vi "Dashboard Main.vi"() -> ()   [LabVIEW 2017]
uses:
  <vilib>/Utility/miscctls.llb/LVRowAndColumnTypeDef.ctl
  <vilib>/event_ctls.llb/eventvkey.ctl
  <vilib>/Rock Robotics/Network Tables/NT Read Boolean.vi
  <vilib>/Rock Robotics/Network Tables/NT Write Boolean.vi
  <vilib>/Rock Robotics/WPI/Dashboard/WPI_DashboardLogging Global.vi
panel:
  out "Camera Image":T1(plugin-control)
  out "Camera Info":cluster{"Mbps LED":bool, "Mbps":dbl, "fps":dbl} {"fps" format="%#.1g"; "Mbps" format="%#.1g"}
  in  "Camera Name":string(combo)="No Camera Selection"
  in  "Camera Settings":T2={"Frame Rate"=30, "Compression"=30, "Size"=1, "DB Camera Config"=FALSE} {"Frame Rate" scale=1.0..30.0; "Compression" scale=100.0..-1.0; "Size" items=["640x480", "320x240", "160x120"]}
  out "Camera Image Right":T1(plugin-control)
  out "NT Connection":bool
  in  "Camera Settings Right":T2={"Frame Rate"=30, "Compression"=30, "Size"=1, "DB Camera Config"=FALSE} {"Frame Rate" scale=1.0..30.0; "Compression" scale=100.0..-1.0; "Size" items=["640x480", "320x240", "160x120"]}
  in  "Camera Name Right":string(combo)="No Camera Selection"
  in  "TCP":refnum<k5>
  in  "Rec Mode":enum32{"Stop", "Record", "Playback"}(radio)
  out "Robot IP":string
  out "Image Message":string="Timeout in Camera Communications"
  in  "Dashboard Tab":T3(tab)
  out "RPED":enum32{"Read", "Write"}(tab)=enum."Write"
  out "Current Left Backward Power":dbl
  out "Current Right Backward Power":dbl
  out "Current Left Forward Power":dbl
  out "Current Right Forward Power":dbl
  in  "Right Backward Power":dbl
  in  "Left Backward Power":dbl
  in  "Right Forward Power":dbl
  in  "Left Forward Power":dbl
  out "Lift":enum32{"Read", "Write"}(tab)=enum."Write"
  out "Current Exchange Encoder Position":dbl
  out "Current Climb Power":dbl
  out "Current Manual Up Power":dbl
  out "Current Manual Down Power":dbl
  out "Current Scale High Encoder Position":dbl
  out "Current Scale Mid Encoder Position":dbl
  out "Current Scale Low Encoder Position":dbl
  out "Current Switch Encoder Position":dbl
  out "Current Stow Encoder Position":dbl
  out "Current Climb Encoder Position":dbl
  out "Current Load Encoder Position":dbl
  out "Current Portal Encoder Position":dbl
  in  "Portal Encoder Position":dbl
  in  "Exchange Encoder Position":dbl
  in  "Climb Power":dbl
  in  "Manual Up Power":dbl
  in  "Manual Down Power":dbl
  in  "Scale High Encoder Position":dbl
  in  "Scale Low Encoder Position":dbl
  in  "Scale Mid Encoder Position":dbl
  in  "Climb Encoder Position":dbl
  in  "Switch Encoder Position":dbl
  in  "Stow Encoder Position":dbl
  in  "Load Encoder Position":dbl
  out "Intake Rotation":enum32{"Read", "Write"}(tab)=enum."Write"
  out "Current Intake Rot Portal Encoder Position":dbl
  out "Current Intake Rot Exchange Encoder Position":dbl
  out "Current Intake Rot Climb Encoder Position":dbl
  out "Current Intake Rot Switch Encoder Position":dbl
  out "Current Intake Rot Stow Encoder Position":dbl
  out "Current Intake Rot Scale High Encoder Position":dbl
  out "Current Intake Rot Load Encoder Position":dbl
  out "Current Intake Rot Manual Down Power":dbl
  out "Current Intake Rot Manual Up Power":dbl
  out "Current Intake Rot Scale Mid Encoder Position":dbl
  out "Current Intake Rot Scale Low Encoder Position":dbl
  in  "Intake Rot Portal Encoder Position":dbl
  in  "Intake Rot Exchange Encoder Position":dbl
  in  "Intake Rot Climb Encoder Positon":dbl
  in  "Intake Rot Switch Encoder Position":dbl
  in  "Intake Rot Stow Encoder Position":dbl
  in  "Intake Rot Scale High Encoder Position":dbl
  in  "Intake Rot Load Encoder Position":dbl
  in  "Intake Rot Manual Up Power":dbl
  in  "Intake Rot Manual Down Power":dbl
  in  "Intake Rot Scale Mid Encoder Position":dbl
  in  "Intake Rot Scale Low Encoder Position":dbl
  out "Drive":enum32{"Read", "Write"}(tab)=enum."Write"
  out "Current Right Low Gear P":dbl
  out "Current Right Low Gear I":dbl
  out "Current Right Low Gear D":dbl
  out "Current Right Low Gear F":dbl
  out "Current Right High Gear I":dbl
  out "Current Right High Gear P":dbl
  out "Current Right High Gear D":dbl
  out "Current Right High Gear F":dbl
  out "Current Left Low Gear P":dbl
  out "Current Left Low Gear I":dbl
  out "Current Left Low Gear D":dbl
  out "Current Left Low Gear F":dbl
  out "Current Left High Gear I":dbl
  out "Current Left High Gear P":dbl
  out "Current Left High Gear D":dbl
  out "Current Left High Gear F":dbl
  in  "Right High Gear F":dbl
  in  "Right High Gear D":dbl
  in  "Right High Gear I":dbl
  in  "Right High Gear P":dbl
  in  "Right  Low Gear F":dbl
  in  "Right Low Gear D":dbl
  in  "Right Low Gear I":dbl
  in  "Right Low Gear P":dbl
  in  "Left High Gear F":dbl
  in  "Left High Gear D":dbl
  in  "Left High Gear I":dbl
  in  "Left High Gear P":dbl
  in  "Left Low Gear F":dbl
  in  "Left Low Gear D":dbl
  in  "Left Low Gear I":dbl
  in  "Left Low Gear P":dbl
  out "Left Wheel":dbl
  out "Right Wheel":dbl
  out "Lift Upper Switch":bool
  out "Arm Lower Switch":bool
  out "IMU":dbl(knob) scale=-360.0..360.0
  out "Last Auto Play Run":string
  out "Brake":bool
  out "Arm":bool
  out "Has Cube":bool
  out "Lift Position":dbl(slide) scale=0.0..7.0
  out "Arm Encoder Position":dbl
  out "Arm Stowed":bool
  out "Lift Stowed":bool
  out "Mode":T4(ring)=enum."Auto Disabled"
  out "Match Time":string="0:00"
  out "High Gear":bool
  out "Lift Encoder Position":dbl
  in  "Override":enum16{"Default", "LL", "LR", "RL", "RR"}(ring)
  in  "RL":T5(ring)
  in  "RR":T6(ring)
  in  "LR":T5(ring)
  in  "LL":T7(ring)
  in  "Position":enum16{"1", "2", "3"}(ring)
  out "Auto":enum32{"Read", "Write"}(tab)
  out "Current Cube PID Acceptable Error":dbl
  out "Current Turning Acceptable Error":dbl
  out "Current Turning Acceptable Tolerance":dbl
  out "Current Number of Loops to be in Tolerance":dbl
  out "Current Number of Loops to be in Acceptable Error":dbl
  out "Current Kp Lower":dbl
  out "Current Kd Lower":dbl
  out "Current Ki Lower":dbl
  out "Current Cube P":dbl
  out "Current Cube D":dbl
  out "Current Cube I":dbl
  out "Current Turn Distance I":dbl
  out "Current Turn Distance P":dbl
  out "Current Kp Upper":dbl
  out "Current Turn Distance D":dbl
  out "Current Kd Upper":dbl
  out "Current Ki Upper":dbl
  in  "Cube PID Acceptable Error":dbl
  in  "Turning Acceptable Error":dbl
  in  "Turning Acceptable Tolerance":dbl
  in  "Number of Loops to be in Acceptable Error":dbl
  in  "Number of Loops to be in Tolerance":dbl
  in  "Kp Lower":dbl
  in  "Ki Lower":dbl
  in  "Kd Lower":dbl
  in  "Turn Distance P":dbl
  in  "Turn Distance I":dbl
  in  "Turn Distance D":dbl
  in  "Kp Upper":dbl
  in  "Ki Upper":dbl
  in  "Kd Upper":dbl
  in  "Cube I":dbl
  in  "Cube D":dbl
  in  "Cube P":dbl
  in  "DB/String 9":string
  in  "DB/String 8":string
  in  "DB/String 7":string
  in  "DB/String 6":string
  in  "DB/String 5":string
  in  "DB/String 4":string
  in  "DB/String 3":string
  in  "DB/String 2":string
  in  "DB/String 1":string
  in  "DB/String 0":string
  in  "DB/Slider 0":dbl(slide) scale=0.0..5.0
  in  "DB/Slider 1":dbl(slide) scale=0.0..5.0
  in  "DB/Slider 2":dbl(slide) scale=0.0..5.0
  in  "DB/Slider 3":dbl(slide) scale=0.0..5.0
  out "DB/LED 3":bool
  out "DB/LED 2":bool
  out "DB/LED 1":bool
  out "DB/LED 0":bool
  in  "DB/Button 3":bool
  in  "DB/Button 2":bool
  in  "DB/Button 1":bool
  in  "DB/Button 0":bool caption="New Name"
  in  "Test Slider":dbl(slide) scale=0.0..100.0 scale format="%#_3g"
  in  "On/Off":bool caption="Solenoid"
  in  "Test Name":u16(ring) items=["Select the test to run..."]
  in  "Test Tree":string(tree)
  in  "Motor":cluster{"Value":dbl, "Enable":bool} {"Value" scale=-1.0..1.0 scale format="%#_3g"}
  out "Progress":T8 {"Test Progress" scale=0.0..100.0}
  in  "Rev/Fwd":cluster{"Forward":bool, "Reverse":bool}
  in  "Test Ring":u16(ring) items=["Monochrome", "Color"]
  out "Cmd Status":string
  in  "Execute Command":bool
  in  "Command Params":string[][](table)
  in  "Command Selection":i32(listbox)
  in  "CheckList":i32(listbox)
  out "Tree":string(tree)
  out "Background":bool
  # "HW"
  # "HW"
  # "Pnuematics"
  # "Turning"
  # "Cube"
  # "Turning"
  # "Cube"
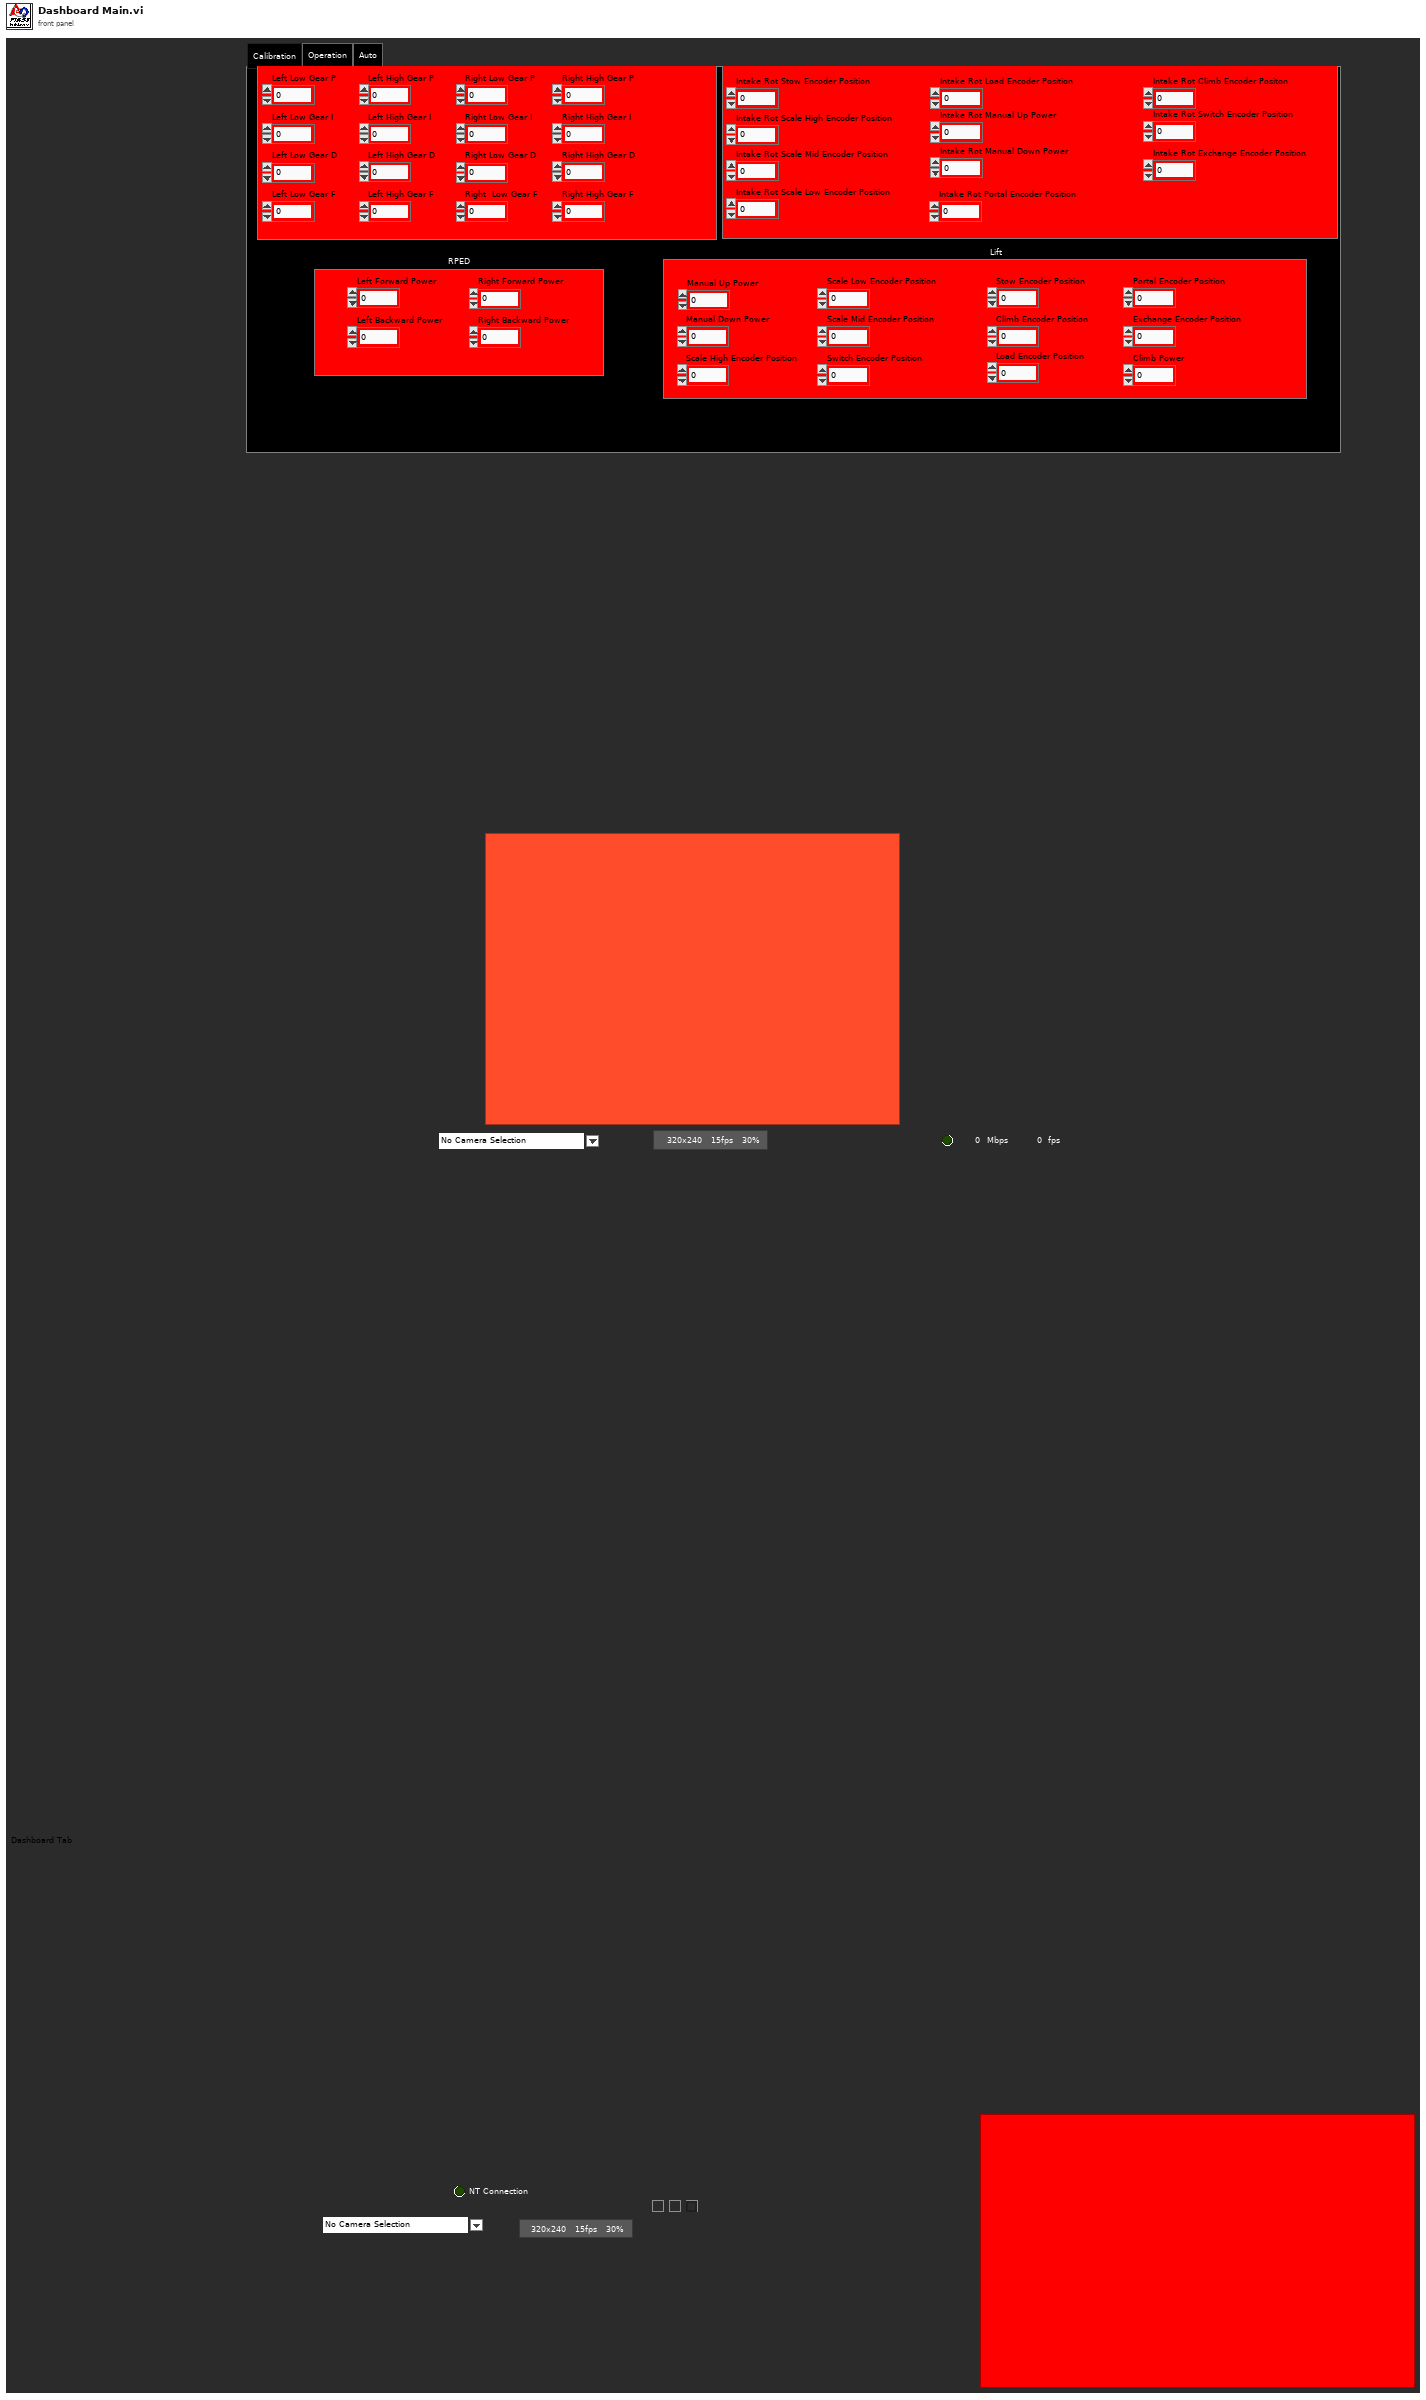
[diagram p1: front panel]
types:
  T1 = typedef "IMAQ Image.ctl" = refnum<image>
  T2 = cluster{"Frame Rate":i32, "Compression":i32, "Size":u16, "DB Camera Config":bool}
  T3 = enum32{"Calibration", "Operation", "Auto", "Basic", "Custom", "Test", "Commands", "Checklist", "Variables"}
  T4 = enum8{"Tele-Op Disabled", "Tele-Op Enabled", "Auto Disabled", "Auto Enabled", "Test Disabled", "Test Enabled", "Disconnected", "No Code", "E-Stop"}
  T5 = enum16{"No_Op", "Auto_Run_Backwards", "Auto_Run_Forwards", "Switch", "Switch_2", "Scale", "Adapt_Scale", "Scale_2", "Switch_Scale", "Scale_Drop_Cube"}
  T6 = enum16{"No_Op", "Auto_Run_Forwards", "Auto_Run_Backwards", "Switch", "Switch_2", "Scale", "Adapt_Scale", "Switch_Scale", "Scale_Switch", "Scale_2", "Drop_Pickup"}
  T7 = enum16{"No_Op", "Auto_Run_Backwards", "Auto_Run_Forwards", "Switch", "Switch_2", "Scale", "Adapt_Scale", "Switch_Scale", "Scale_Switch", "Scale_2", "Drop_Pickup"}
  T8 = cluster{"Test Progress":u8, "Test Progress Text":string}
  T9 = cluster{"Save Path":path, "Interval (s)":dbl, "Keep":i32}
  T10 = enum32{"Drive", "Camera", "Basic", "Custom", "Test", "Commands", "Checklist", "Variables"}
  T11 = typedef "Image Type" = u32
  T12 = cluster{"IDs":cluster{"RPC field ID":u16, "Unique ID":u16}, "String":string}
  T13 = cluster{"Error Strings":string, "Disable Counts":cluster{u16, u16}, "Rail Faults":cluster{u16, u16, u16}, "Robot IP":string, "DB Mode":u8, "Event Info":cluster{"Name":string, "Type":u8, "Number":u16, "Replay":u8}}
  T14 = cluster{"Storage":cluster{"Disk Free":u64, "RAM Block":u32, "RAM free":u32}, "CPU Utilization":cluster{"CPU % ISR":sgl, "CPU % Time Crit":sgl, "CPU % Timed Str":sgl, "CPU % High":sgl, "CPU % Above":sgl, "CPU % Normal":sgl, "CPU % Low":sgl}, "CAN":cluster{"% Bus Utilization":sgl, "Bus Off Cnt":u32, "TX_FIFO Full Cnt":u32, "Receive Error Cnt":u8, "Transmit Error Cnt":u8}, "HID":cluster{"HID Outputs":u32, "Rumble Low":u16, "Rumble High":u16}[]}
  T15 = cluster{"Status bits":cluster{"Test Mode":bool, "Autonomous":bool, "Enabled":bool, "Code Start":bool, "Brownout":bool, "Reserved 2":bool, "Reserved 3":bool, "E-Stop":bool}, "Code Trace":cluster{"Disabled":bool, "TeleOp":bool, "Auto":bool, "Test":bool}, "Controller Type":enum16{"unknown", "cRIO", "roboRio"}, "Code?":enum16{"unknown", "noCode", "code"}, "Battery V":dbl}
  T16 = cluster{"Control Bits":cluster{"TestMode":bool, "Autonomous":bool, "Enabled":bool, "FMS Present":bool, bool, bool, bool, "E-Stop":bool}, "Team Station ":u8, "Countdown":sgl, "Joystick Values":cluster{"Axes":dbl[], "Buttons":bool[], "POVs":i16[]}[]}
  T17 = cluster{"Camera Image":refnum<vi>, "Dashboard Tab":refnum<vi>, "Background":refnum<vi>, "Rec Mode":refnum<vi>, "Test Slider":refnum<vi>, "On/Off ":refnum<vi>, "Test Ring":refnum<vi>, "Rev/Fwd":refnum<vi>, "Test Name":refnum<vi>, "Motor":refnum<vi>, "Progress":refnum<vi>, "CheckList":refnum<vi>, "Tree":refnum<vi>, "Test Tree":refnum<vi>, "Command Params":refnum<vi>, "Command Selection":refnum<vi>, "Execute Command":refnum<vi>, "Cmd Status":refnum<vi>, "Camera Settings":refnum<vi>, "Camera Name":refnum<vi>, "Camera Info":refnum<vi>, "Camera Settings Right":refnum<vi>, "Camera Name Right":refnum<vi>, "Camera Image Right":refnum<vi>}
  T18 = cluster{"Camera Name Right":string, string, "Saved DB Images Info":cluster{"Save Path":path, "Interval (s)":dbl, "Keep":i32}}
  T19 = cluster{"Camera Name":string, string, "Saved DB Images Info":cluster{"Save Path":path, "Interval (s)":dbl, "Keep":i32}}
  T20 = cluster{"Operation":enum16{"Update", "Clear"}, "Color Box":u32}[]
  T21 = typedef "eventvkey.ctl" = enum16{"ASCII", "Enter", "Return", "Shift", "Ctrl", "Alt", "Cmd", "Opt", "Caps", "NumLock", "Clear", "Break", "Up", "Down", "Left", "Right", "Insert", "Delete", "Home", "End", "PageUp", "PageDown", "Escape", "Help", "Pause", "ScrollLock", "F1", "F2", "F3", "F4", "F5", "F6", "F7", "F8", "F9", "F10", "F11", "F12", "F13", "F14", "F15", "F16", "F17", "F18", "F19", "F20", "F21", "F22", "F23", "F24", "Play", "VolumeUp", "VolumeDown", "Mute", "Two Byte Char"}
  T22 = cluster{"Image Size":bool, "Image Type":bool, "Pixel Value":bool, "ROI Information":bool, "Zoom Factor":bool}
  T23 = cluster{"Operation":enum16{"Update", "Clear"}, "Color Box":u32}
  T24 = typedef "LVRowAndColumnTypeDef.ctl" = cluster{"Row":i32, "Column":i32}
  T25 = cluster{"Shift":bool, "Ctrl":bool, "Alt":bool, "Cmd":bool, "Opt":bool}
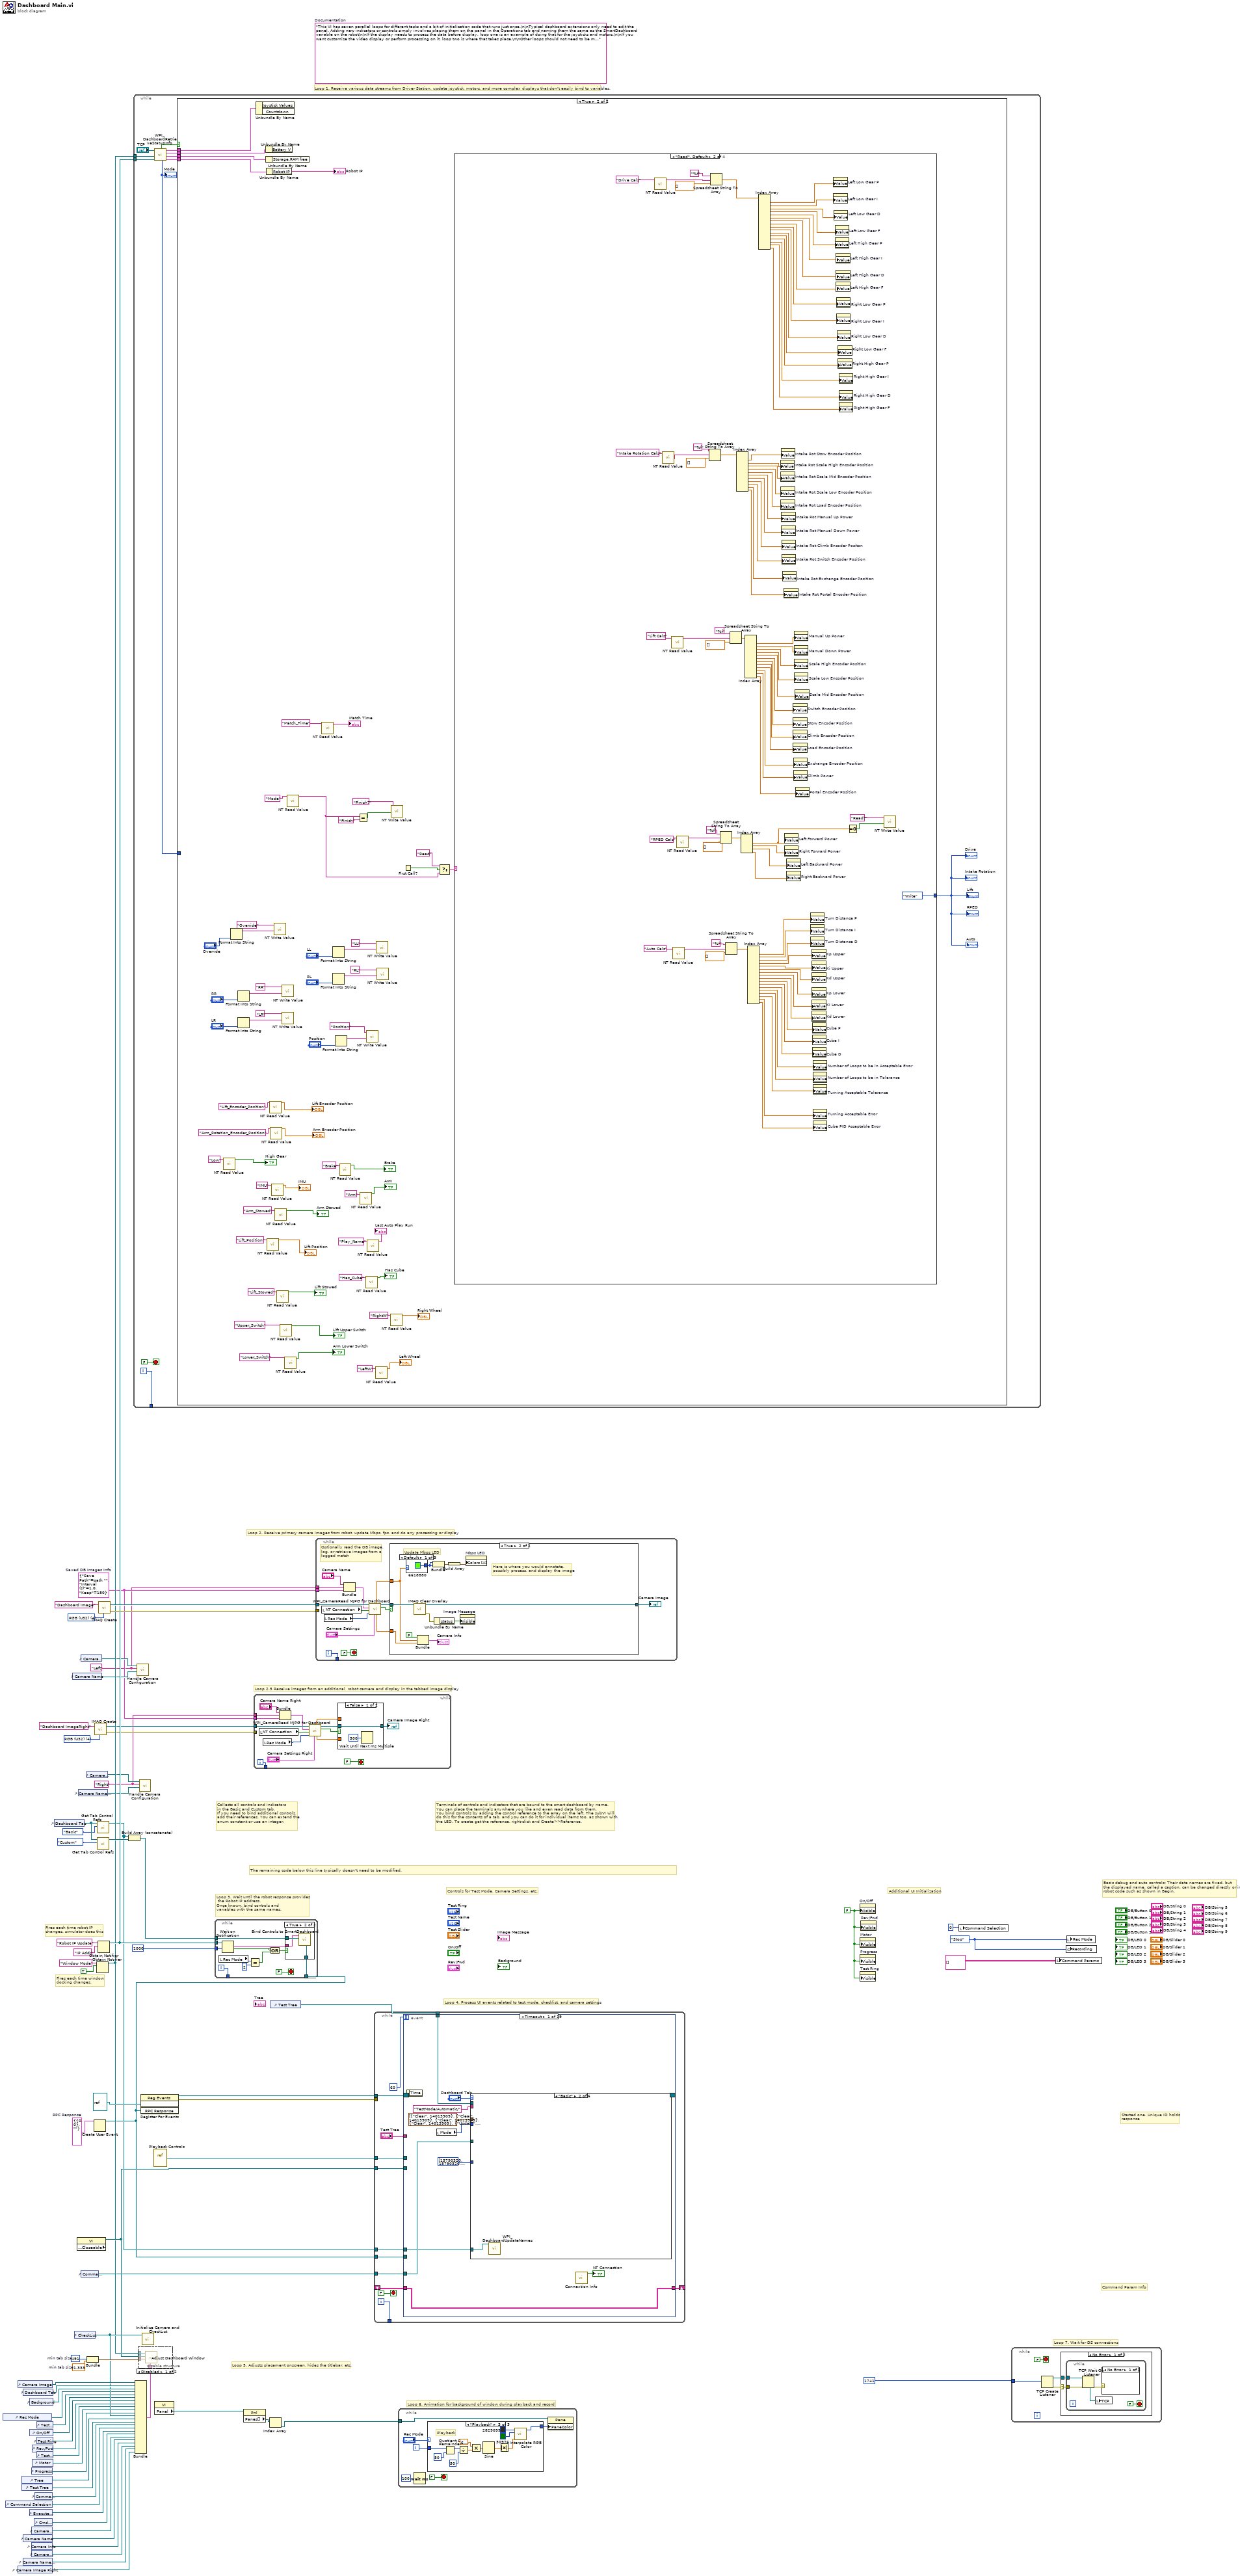
[diagram p0: block diagram]
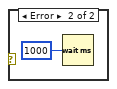
[diagram p4: hidden frame]
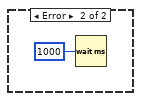
[diagram p5: hidden frame]
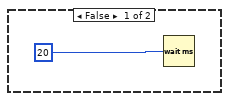
[diagram p6: hidden frame]
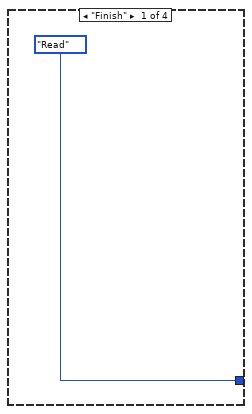
[diagram p7: hidden frame]
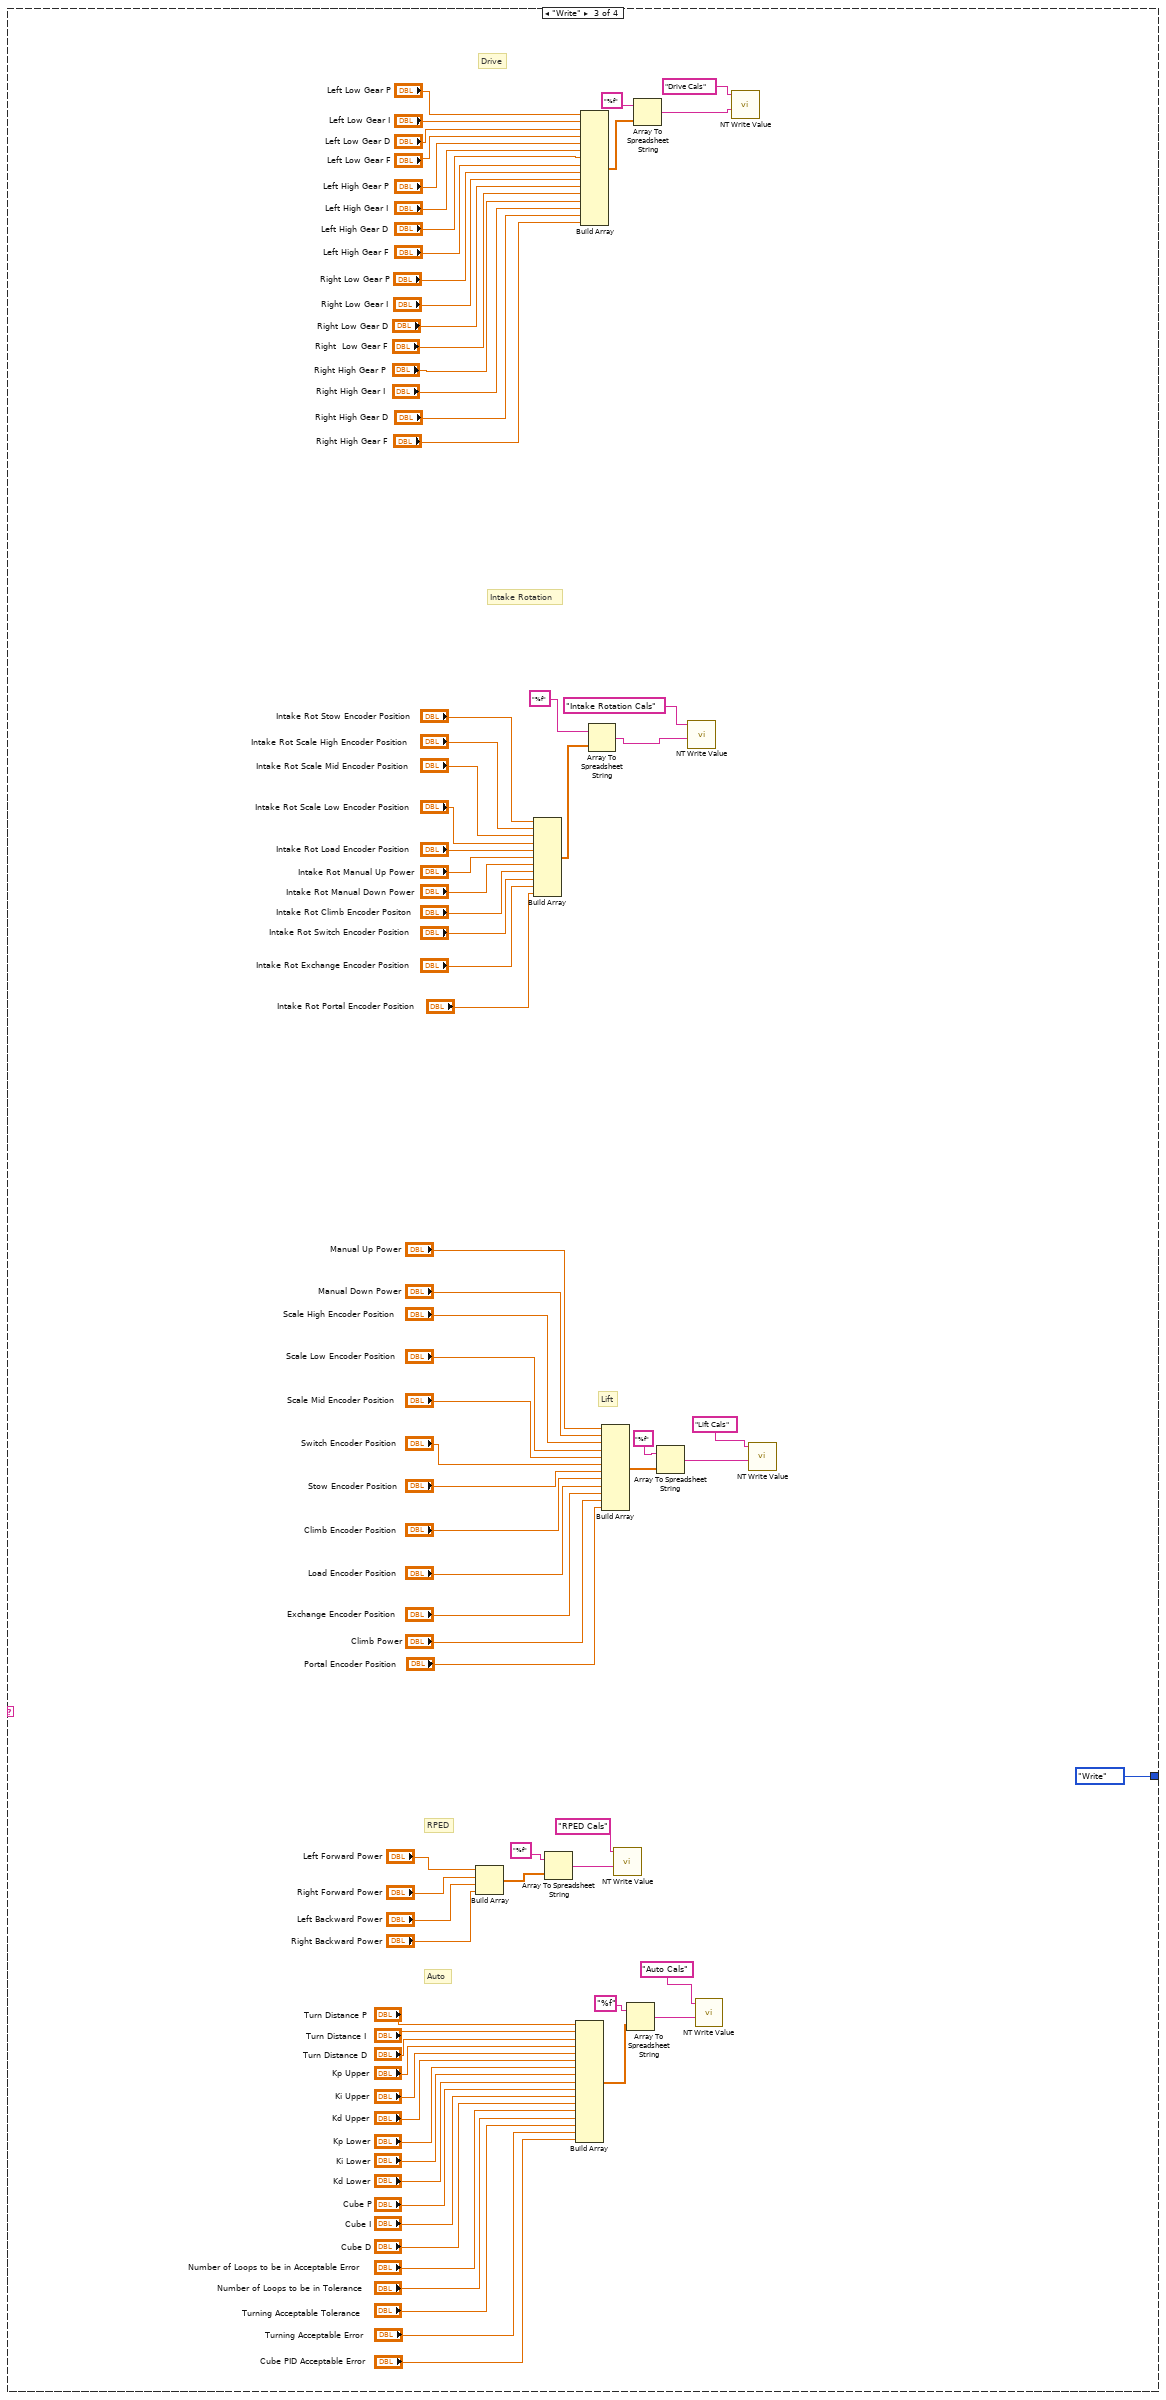
[diagram p8: hidden frame]
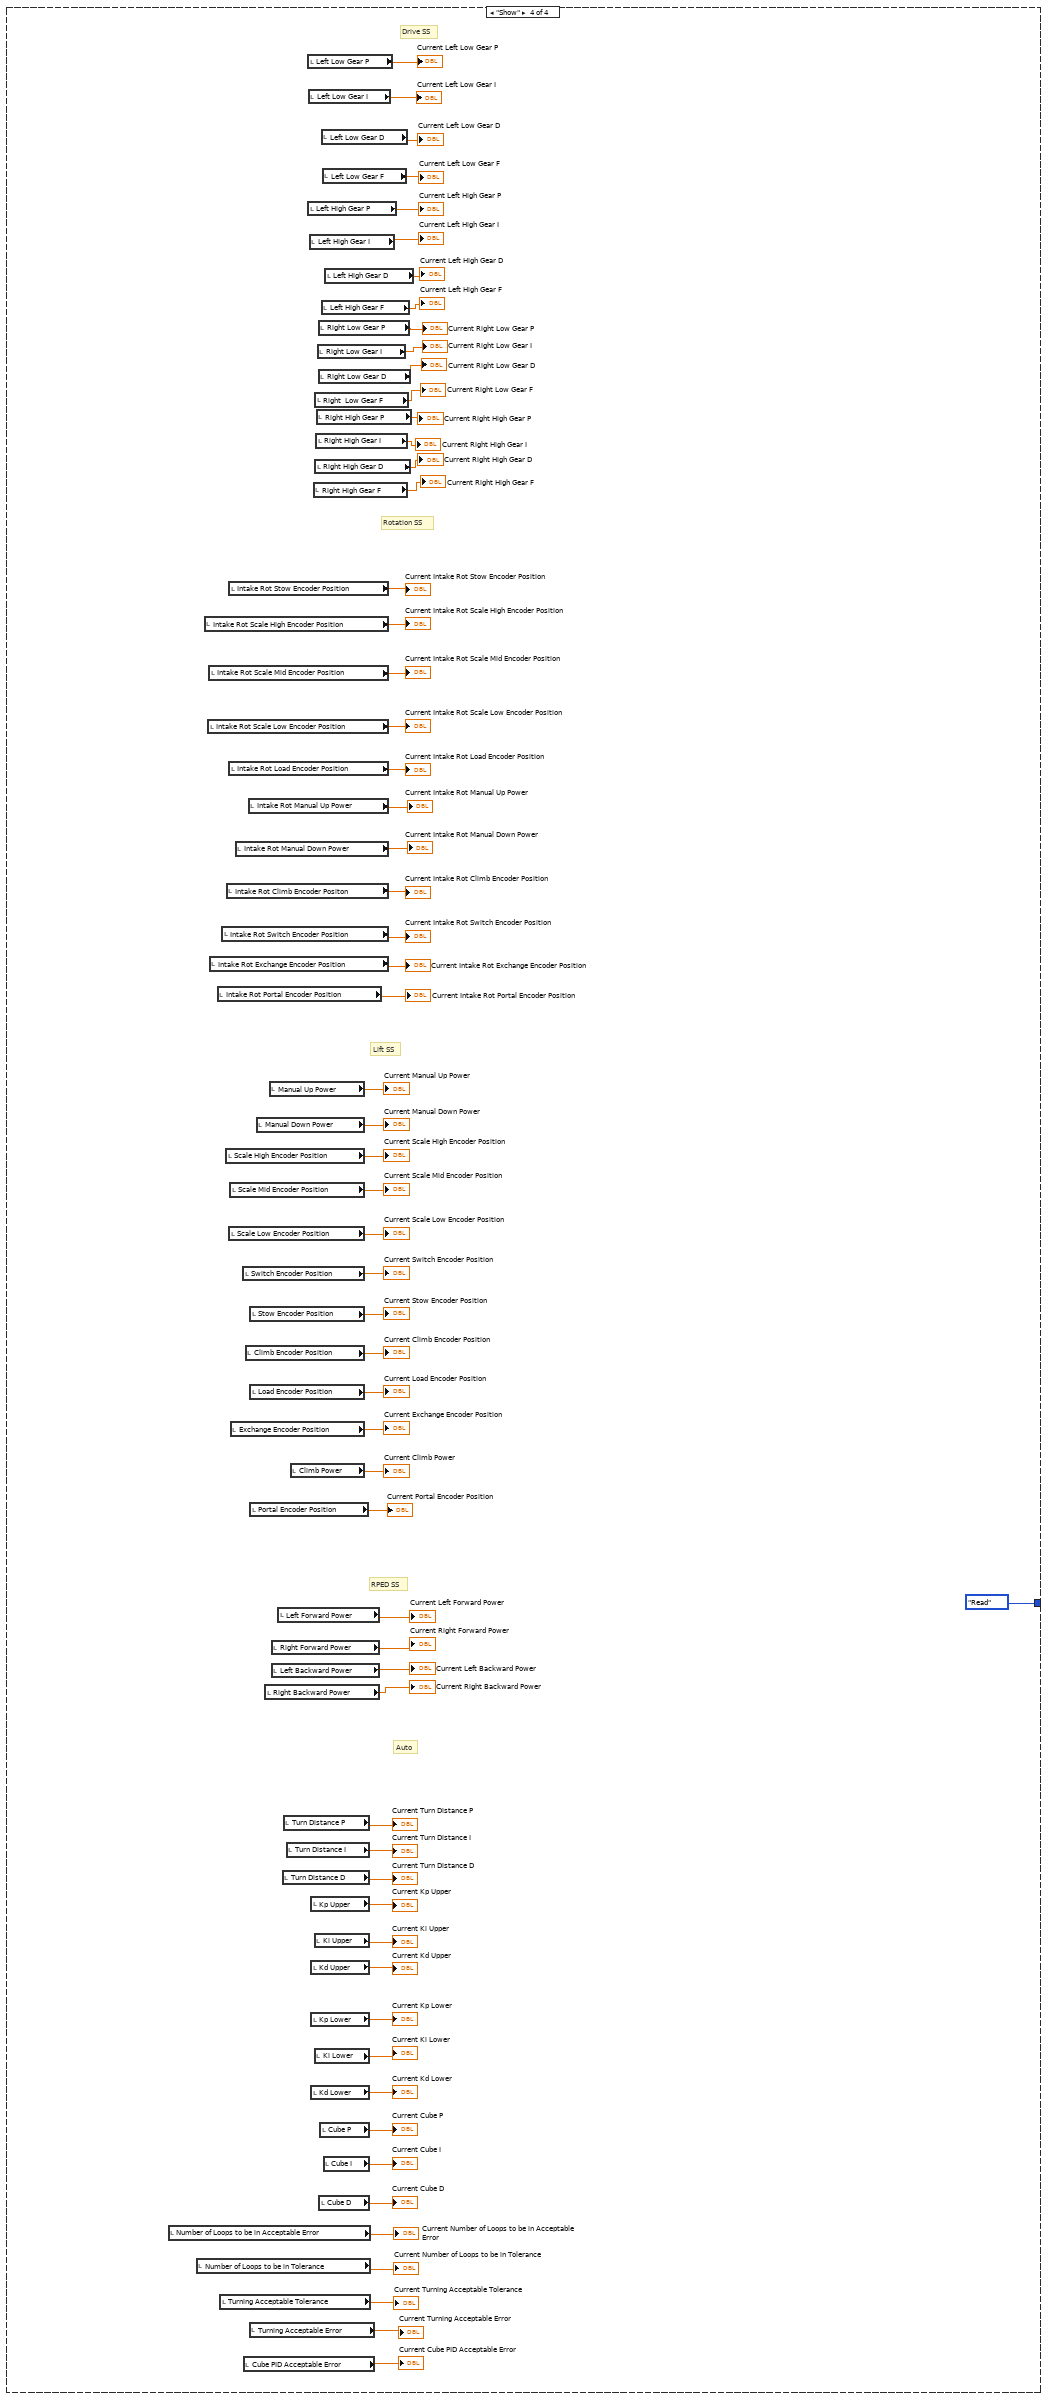
[diagram p9: hidden frame]
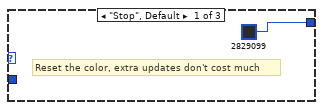
[diagram p10: hidden frame]
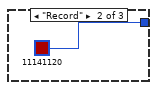
[diagram p11: hidden frame]
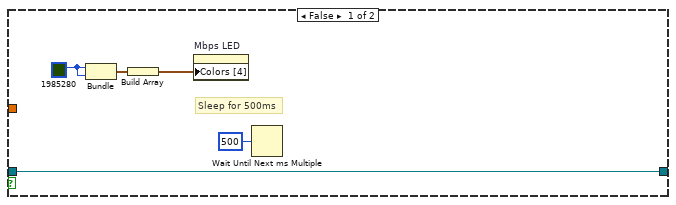
[diagram p13: hidden frame]
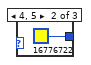
[diagram p14: hidden frame]
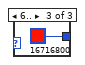
[diagram p15: hidden frame]
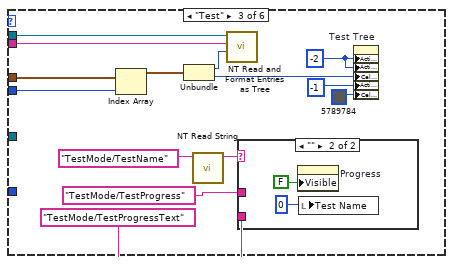
[diagram p17: hidden frame]
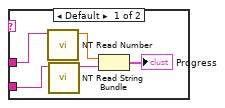
[diagram p18: hidden frame]
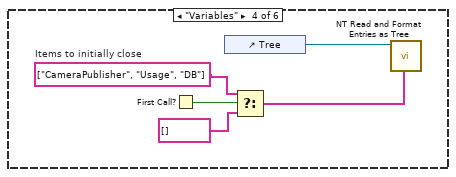
[diagram p19: hidden frame]
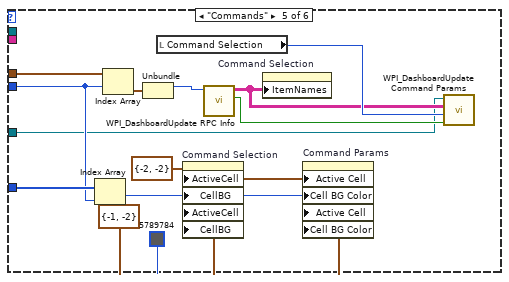
[diagram p20: hidden frame]
diagram:
  w3 = T9 {"Save Path"=path "", "Interval (s)"=1.0, "Keep"=180}  # Saved DB Images Info
  w2 = "Right"
  w1 = "Left"
  w13 = T11 4 items=["Grayscale (U8)", "Grayscale (I16)", "Grayscale (SGL)", "Complex (CSG)", "RGB (U32)", "HSL (U32)", "RGB (U64)"] ("Image Type")
  w27 = T12 {"IDs"={"RPC field ID"=0, "Unique ID"=0}, "String"=""}  # RPC Response
  w49 = 491  # min tab size
  w48 = 1.333  # min tab size
  w56 = enum32{"Stop", "Record", "Playback"}."Stop" ("Rec Mode")
  w33 = FALSE ("Visible")
  (unwired) "This VI has seven parallel loops for different tasks and a bit of initialization code that runs just once.\n\nTypical dashboard extensions only need to edit the panel. Adding new indicators or controls simply involves placing them on the panel in the Operations tab and naming them the same as the SmartDashboard variable on the robot\n\nIf the display needs to process the data before display, loop one is an example of doing that for the joysticks and motors.\n\nIf you want customize the video display or perform processing on it, loop two is where that takes place.\n\nOther loops should not need to be modified. They are pretty standard, and document the task they perform."  # Documentation
  w73 = T11 4 items=["Grayscale (U8)", "Grayscale (I16)", "Grayscale (SGL)", "Complex (CSG)", "RGB (U32)", "HSL (U32)", "RGB (U64)"] ("Image Type")
  # "Loop 5. Adjusts placement onscreen, hides the titlebar, etc."
  # "Loop 2.5 Receive images from an additional  robot camera and display in the tabbed image display"
  # "Command Param Info"
  # "Started one, Unique ID holds\nresponse"
  # "Loop 7. Wait for DS connections"
  # "Basic debug and auto controls: Their data names are fixed, but\nthe displayed name, called a caption, can be changed directly or in\nrobot code such as shown in Begin."
  # "Controls for Test Mode, Camera Settings, etc."
  # "Additional UI Initialization"
  # "Loop 6. Animation for background of window during playback and record"
  # "Fires each time robot IP\nchanges, simulator does this"
  # "Fires each time window\ndocking changes."
  # "Collects all controls and indicators\nin the Basic and Custom tab.\nIf you need to bind additional controls,\nadd their references. You can extend the\nenum constant or use an integer."
  # "The remaining code below this line typically doesn't need to be modified."
  # "Loop 4. Process UI events related to test mode, checklist, and camera settings"
  # "Terminals of controls and indicators that are bound to the smart dashboard by name.\nYou can place the terminals anywhere you like and even read data from them.\nYou bind controls by adding the control reference to the array on the left. The subVI will\ndo this for the contents of a tab, and you can do it for individual items too, as shown with\nthe LED. To create get the reference, right-click and Create>>Reference."
  # "Loop 3. Wait until the robot response provides\n the Robot IP address.\nOnce known, bind controls and\nvariables with the same names."
  # "Loop 1. Receive various data streams from Driver Station, update joystick, motors, and more complex displays that don't easily bind to variables."
  # "Loop 2. Receive primary camera images from robot, update Mbps, fps, and do any processing or display"
  n1 = control-ref of="Rec Mode"() -> (w39:refnum<vi>)
  n2 = control-ref of="Command Selection"() -> (w26:refnum<vi>)
  n3 = control-ref of="Camera Image Right"() -> (w6:refnum<vi>)
  n4 = control-ref of="Camera Image"() -> (w51:refnum<vi>)
  n5 = control-ref of="Tree"() -> (w43:refnum<vi>)
  n6 = control-ref of="Test Tree"() -> (w42:refnum<vi>)
  n7 = control-ref of="Dashboard Tab"() -> (w50:refnum<vi>)
  n8 = control-ref of="Camera Name"() -> (w17:refnum<vi>)
  n9 = control-ref of="Camera Name Right"() -> (w7:refnum<vi>)
  n10 = control-ref of="Execute Command"() -> (w28:refnum<vi>)
  n11 = control-ref of="Background"() -> (w46:refnum<vi>)
  n12 = control-ref of="On/Off"() -> (w37:refnum<vi>)
  n13 = control-ref of="Progress"() -> (w34:refnum<vi>)
  n14 = control-ref of="Camera Settings"() -> (w18:refnum<vi>)
  n15 = control-ref of="Camera Info"() -> (w16:refnum<vi>)
  n16 = control-ref of="Camera Settings Right"() -> (w8:refnum<vi>)
  n17 = control-ref of="Rev/Fwd"() -> (w35:refnum<vi>)
  n18 = control-ref of="Motor"() -> (w40:refnum<vi>)
  n19 = control-ref of="Cmd Status"() -> (w22:refnum<vi>)
  n20 = control-ref of="Command Params"() -> (w29:refnum<vi>)
  n21 = control-ref of="Test Slider"() -> (w38:refnum<vi>)
  n22 = control-ref of="Test Ring"() -> (w36:refnum<vi>)
  n23 = control-ref of="Test Name"() -> (w41:refnum<vi>)
  n24 = control-ref of="Dashboard Tab"() -> (w54:refnum<vi>)
  n25 = control-ref of="Camera Name"() -> (w19:refnum<vi>)
  n26 = control-ref of="CheckList"() -> (w44:refnum<vi>)
  n27 = property class="VI" props=["Front Panel.Closeable"]() -> (reference out=w55:refnum<vi>)  [unwired: 2 in, 2 out]
  n28 = control-ref of="Camera Name Right"() -> (w9:refnum<vi>)
  n29 = control-ref of="Camera Settings"() -> (w20:refnum<vi>)
  n30 = control-ref of="Command Params"() -> (w21:refnum<vi>)
  n31 = control-ref of="Camera Settings Right"() -> (w10:refnum<vi>)
  n32 = Bundle("min tab size"=w49, "min tab size"=w48) -> (w47:cluster{"min tab size":i32, "min tab size":dbl})  [unwired: 1 in]
  n33 = Create User Event(user event datatype=w27) -> (user event=w23:refnum<user-event>)  [unwired: 1 in, 1 out]
  n34 = call "IMAQ Create"("Image Name"="Dashboard ImageRight", "Image Type"=w13) -> ("New Image"=w12:T1, "error out"=w11:errorcluster)  [unwired: 2 in, 1 out]
  n35 = Obtain Notifier(name (unnamed)="Window Mode", notification data type=TRUE) -> (notifier out=w31:refnum<notifier>)  [unwired: 2 in, 2 out]
  n36 = call <vilib>:"Get Tab Control Refs.vi"("Page Index"=T10."Basic" ("Dashboard Tab"), "TabControl in"=w54) -> ("ControlsOnPage"=w15:refnum<vi>[])  [unwired: 9 in]
  n37 = call <vilib>:"Get Tab Control Refs.vi"("Page Index"=T10."Custom" ("Dashboard Tab"), "TabControl in"=w54) -> ("ControlsOnPage"=w53:refnum<vi>[])  [unwired: 9 in]
  n38 = Obtain Notifier(name (unnamed)="Robot IP Update", notification data type="IP Addr" ("name (unnamed)")) -> (notifier out=w32:refnum<notifier>)  [unwired: 2 in, 2 out]
  n39 = call "IMAQ Create"("Image Name"="Dashboard Image", "Image Type"=w73) -> ("New Image"=w71:T1, "error out"=w70:errorcluster)  [unwired: 2 in, 1 out]
  n40 = Build Array (concatenate)(w15, w53) -> (w52:refnum<vi>[])
  n41 = while {
    tunnel: [w83] -> _
    tunnel: w32 -> [w77]
    tunnel: w31 -> [w74]
    i -> [w83]
    stop <- FALSE stop-if-true
    n42 = call <vilib>:"WPI_DashboardRetrieveStatusInfo.vi"("Binding Refnum"=w77, "Window Mode Notifier"=w74, "TCP Cnx"="TCP") -> ("Power and Errors"=w78:T13, "Robot Metrics"=w81:T14, "Status Info"=w82:T15, "Control Info"=w79:T16, "Robot Mode"=w76:T4, "Process?"=w80:bool)  [unwired: 3 in]
    "Mode" <- w76
    n43 = case shown="True" w80 {
      tunnel: w82 -> [_ w149]
      tunnel: w81 -> [_ w148]
      tunnel: w79 -> [_ w147]
      tunnel: w78 -> [_ w146]
      tunnel: w76 -> [_ _]
      frame False {
        n44 = Wait (ms)(milliseconds to wait=u32 20) -> ()  [unwired: 1 out]
      }
      frame True {
        n45 = call-poly <vilib>:"NT Read Value.vi"("Name"="Low") -> ("Boolean"=→"High Gear":bool)  [unwired: 9 in, 1 out]
        n46 = Format Into String("Override") -> (resulting string=w100:string)  [unwired: 3 in, 1 out]
        n47 = Format Into String("RR") -> (resulting string=w111:string)  [unwired: 3 in, 1 out]
        n48 = Format Into String("LR") -> (resulting string=w110:string)  [unwired: 3 in, 1 out]
        n49 = Unbundle By Name(w147) -> ()  [unwired: 2 out]
        n50 = Unbundle By Name(w149) -> ()  [unwired: 1 out]
        n51 = Unbundle By Name(w148) -> ()  [unwired: 1 out]
        n52 = Unbundle By Name(w146) -> ("Robot IP"=→"Robot IP":string)
        n53 = call-poly <vilib>:"NT Read Value.vi"("Name"="Lift_Position") -> ("Numeric"=→"Lift Position":dbl)  [unwired: 9 in, 1 out]
        n54 = call-poly <vilib>:"NT Read Value.vi"("Name"="Lift_Encoder_Position") -> ("Numeric"=→"Lift Encoder Position":dbl)  [unwired: 9 in, 1 out]
        n55 = call-poly <vilib>:"NT Read Value.vi"("Name"="Arm_Rotation_Encoder_Position") -> ("Numeric"=→"Arm Encoder Position":dbl)  [unwired: 9 in, 1 out]
        n56 = call-poly <vilib>:"NT Read Value.vi"("Name"="IMU") -> ("Numeric"=→"IMU":dbl)  [unwired: 9 in, 1 out]
        n57 = call-poly <vilib>:"NT Write Value.vi"("String"=w100, "Name"="Override") -> ()  [unwired: 9 in, 1 out]
        n58 = call-poly <vilib>:"NT Read Value.vi"("Name"="Arm_Stowed") -> ("Boolean"=→"Arm Stowed":bool)  [unwired: 9 in, 1 out]
        n59 = call-poly <vilib>:"NT Read Value.vi"("Name"="Lift_Stowed") -> ("Boolean"=→"Lift Stowed":bool)  [unwired: 9 in, 1 out]
        n60 = call-poly <vilib>:"NT Read Value.vi"("Name"="Upper_Switch") -> ("Boolean"=→"Lift Upper Switch":bool)  [unwired: 9 in, 1 out]
        n61 = call-poly <vilib>:"NT Write Value.vi"("String"=w110, "Name"="LR") -> ()  [unwired: 9 in, 1 out]
        n62 = call-poly <vilib>:"NT Write Value.vi"("String"=w111, "Name"="RR") -> ()  [unwired: 9 in, 1 out]
        n63 = call-poly <vilib>:"NT Read Value.vi"("Name"="Lower_Switch") -> ("Boolean"=→"Arm Lower Switch":bool)  [unwired: 9 in, 1 out]
        n64 = call-poly <vilib>:"NT Read Value.vi"("Name"="Mode") -> ("String"=w94:string)  [unwired: 9 in, 1 out]
        n65 = call-poly <vilib>:"NT Read Value.vi"("Name"="Match_Time") -> ("String"=→"Match Time":string)  [unwired: 9 in, 1 out]
        n66 = Format Into String("LL") -> (resulting string=w115:string)  [unwired: 3 in, 1 out]
        n67 = Format Into String("RL") -> (resulting string=w114:string)  [unwired: 3 in, 1 out]
        n68 = Format Into String("Position") -> (resulting string=w117:string)  [unwired: 3 in, 1 out]
        n69 = call-poly <vilib>:"NT Read Value.vi"("Name"="Brake") -> ("Boolean"=→"Brake":bool)  [unwired: 9 in, 1 out]
        n70 = Equal?(x=w94, y="Finish") -> (x = y?=w131:bool)
        n71 = call-poly <vilib>:"NT Read Value.vi"("Name"="Arm") -> ("Boolean"=→"Arm":bool)  [unwired: 9 in, 1 out]
        n72 = call-poly <vilib>:"NT Read Value.vi"("Name"="Has_Cube") -> ("Boolean"=→"Has Cube":bool)  [unwired: 9 in, 1 out]
        n73 = call-poly <vilib>:"NT Write Value.vi"("String"=w117, "Name"="Position") -> ()  [unwired: 9 in, 1 out]
        n74 = call-poly <vilib>:"NT Read Value.vi"("Name"="Play_Name") -> ("String"=→"Last Auto Play Run":string)  [unwired: 9 in, 1 out]
        n75 = call-poly <vilib>:"NT Read Value.vi"("Name"="LeftW") -> ("Numeric"=→"Left Wheel":dbl)  [unwired: 9 in, 1 out]
        n76 = call-poly <vilib>:"NT Write Value.vi"("String"=w115, "Name"="LL") -> ()  [unwired: 9 in, 1 out]
        n77 = call-poly <vilib>:"NT Write Value.vi"("String"=w114, "Name"="RL") -> ()  [unwired: 9 in, 1 out]
        n78 = call-poly <vilib>:"NT Read Value.vi"("Name"="RightW") -> ("Numeric"=→"Right Wheel":dbl)  [unwired: 9 in, 1 out]
        n79 = call-poly <vilib>:"NT Write Value.vi"("Boolean"=w131, "Name"="Finish?") -> ()  [unwired: 9 in, 1 out]
        n80 = First Call?() -> (First Call?: T/F=w96:bool)
        n81 = Select(t="Read" ("f"), s=w96, f=w94) -> (s? t:f=w97:string)
        n82 = case shown="\"Read\", Default" w97 {
          tunnel: [enum32{"Read", "Write"}."Read" ("Drive") enum32{"Read", "Write"}."Write" ("Drive") enum32{"Read", "Write"}."Write" ("Drive") enum32{"Read", "Write"}."Read" ("Drive")] -> w141
          frame "Finish" {
          }
          frame "Read", Default {
            n83 = call-poly <vilib>:"NT Read Value.vi"("Name"="Drive Cals") -> ("String"=w222:string)  [unwired: 9 in, 1 out]
            n84 = call-poly <vilib>:"NT Read Value.vi"("Name"="Intake Rotation Cals") -> ("String"=w221:string)  [unwired: 9 in, 1 out]
            n85 = call-poly <vilib>:"NT Read Value.vi"("Name"="Lift Cals") -> ("String"=w220:string)  [unwired: 9 in, 1 out]
            n86 = call-poly <vilib>:"NT Read Value.vi"("Name"="Auto Cals") -> ("String"=w205:string)  [unwired: 9 in, 1 out]
            n87 = call-poly <vilib>:"NT Read Value.vi"("Name"="RPED Cals") -> ("String"=w219:string)  [unwired: 9 in, 1 out]
            n88 = Spreadsheet String To Array(format string="%f", spreadsheet string=w221, array type (2D Dbl)=dbl[] []) -> (array=w234:dbl[])  [unwired: 1 in]
            n89 = Spreadsheet String To Array(format string="%f", spreadsheet string=w222, array type (2D Dbl)=dbl[] []) -> (array=w237:dbl[])  [unwired: 1 in]
            n90 = Spreadsheet String To Array(format string="%f", spreadsheet string=w219, array type (2D Dbl)=dbl[] []) -> (array=w230:dbl[])  [unwired: 1 in]
            n91 = Spreadsheet String To Array(format string="%f", spreadsheet string=w205, array type (2D Dbl)=dbl[] []) -> (array=w202:dbl[])  [unwired: 1 in]
            n92 = Spreadsheet String To Array(format string="%f", spreadsheet string=w220, array type (2D Dbl)=dbl[] []) -> (array=w232:dbl[])  [unwired: 1 in]
            n93 = Index Array(array=w234) -> (element #1=w217:dbl, element #2=w182:dbl, element #3=w194:dbl, element #4=w193:dbl, element #5=w192:dbl, element #6=w191:dbl, element #7=w190:dbl, element #8=w189:dbl, element #9=w188:dbl, element #10=w183:dbl, element #11=w151:dbl)  [unwired: 11 in]
            n94 = Index Array(array=w230) -> (element #1=w164:dbl, element #2=w227:dbl, element #3=w187:dbl, element #4=w186:dbl)  [unwired: 4 in]
            n95 = Index Array(array=w232) -> (element #1=w216:dbl, element #2=w215:dbl, element #3=w185:dbl, element #4=w184:dbl, element #5=w172:dbl, element #6=w171:dbl, element #7=w170:dbl, element #8=w169:dbl, element #9=w168:dbl, element #10=w167:dbl, element #11=w166:dbl, element #12=w152:dbl)  [unwired: 12 in]
            n96 = Index Array(array=w202) -> (element #1=w200:dbl, element #2=w199:dbl, element #3=w198:dbl, element #4=w197:dbl, element #5=w196:dbl, element #6=w195:dbl, element #7=w178:dbl, element #8=w177:dbl, element #9=w176:dbl, element #10=w179:dbl, element #11=w180:dbl, element #12=w181:dbl, element #13=w175:dbl, element #14=w174:dbl, element #15=w173:dbl, element #16=w162:dbl, element #17=w161:dbl)  [unwired: 17 in]
            n97 = Index Array(array=w237) -> (element #1=w213:dbl, element #2=w212:dbl, element #3=w211:dbl, element #4=w210:dbl, element #5=w209:dbl, element #6=w208:dbl, element #7=w207:dbl, element #8=w206:dbl, element #9=w160:dbl, element #10=w159:dbl, element #11=w158:dbl, element #12=w157:dbl, element #13=w156:dbl, element #14=w155:dbl, element #15=w154:dbl, element #16=w153:dbl)  [unwired: 16 in]
            n98 = property on="Intake Rot Scale High Encoder Position" class="DigNum (strict)"("Value"=w182) -> ()  [unwired: 2 in, 2 out]
            n99 = property on="Intake Rot Scale Mid Encoder Position" class="DigNum (strict)"("Value"=w194) -> ()  [unwired: 2 in, 2 out]
            n100 = property on="Intake Rot Scale Low Encoder Position" class="DigNum (strict)"("Value"=w193) -> ()  [unwired: 2 in, 2 out]
            n101 = property on="Intake Rot Load Encoder Position" class="DigNum (strict)"("Value"=w192) -> ()  [unwired: 2 in, 2 out]
            n102 = property on="Intake Rot Stow Encoder Position" class="DigNum (strict)"("Value"=w217) -> ()  [unwired: 2 in, 2 out]
            n103 = property on="Intake Rot Manual Up Power" class="DigNum (strict)"("Value"=w191) -> ()  [unwired: 2 in, 2 out]
            n104 = property on="Intake Rot Manual Down Power" class="DigNum (strict)"("Value"=w190) -> ()  [unwired: 2 in, 2 out]
            n105 = property on="Intake Rot Climb Encoder Positon" class="DigNum (strict)"("Value"=w189) -> ()  [unwired: 2 in, 2 out]
            n106 = property on="Intake Rot Switch Encoder Position" class="DigNum (strict)"("Value"=w188) -> ()  [unwired: 2 in, 2 out]
            n107 = property on="Intake Rot Exchange Encoder Position" class="DigNum (strict)"("Value"=w183) -> ()  [unwired: 2 in, 2 out]
            n108 = property on="Intake Rot Portal Encoder Position" class="DigNum (strict)"("Value"=w151) -> ()  [unwired: 2 in, 2 out]
            n109 = property on="Left Forward Power" class="DigNum (strict)"("Value"=w164) -> ()  [unwired: 2 in, 2 out]
            n110 = property on="Right Forward Power" class="DigNum (strict)"("Value"=w227) -> ()  [unwired: 2 in, 2 out]
            n111 = property on="Left Backward Power" class="DigNum (strict)"("Value"=w187) -> ()  [unwired: 2 in, 2 out]
            n112 = property on="Right Backward Power" class="DigNum (strict)"("Value"=w186) -> ()  [unwired: 2 in, 2 out]
            n113 = property on="Switch Encoder Position" class="DigNum (strict)"("Value"=w171) -> ()  [unwired: 2 in, 2 out]
            n114 = property on="Stow Encoder Position" class="DigNum (strict)"("Value"=w170) -> ()  [unwired: 2 in, 2 out]
            n115 = property on="Climb Encoder Position" class="DigNum (strict)"("Value"=w169) -> ()  [unwired: 2 in, 2 out]
            n116 = property on="Load Encoder Position" class="DigNum (strict)"("Value"=w168) -> ()  [unwired: 2 in, 2 out]
            n117 = property on="Exchange Encoder Position" class="DigNum (strict)"("Value"=w167) -> ()  [unwired: 2 in, 2 out]
            n118 = property on="Climb Power" class="DigNum (strict)"("Value"=w166) -> ()  [unwired: 2 in, 2 out]
            n119 = property on="Manual Up Power" class="DigNum (strict)"("Value"=w216) -> ()  [unwired: 2 in, 2 out]
            n120 = property on="Manual Down Power" class="DigNum (strict)"("Value"=w215) -> ()  [unwired: 2 in, 2 out]
            n121 = property on="Scale High Encoder Position" class="DigNum (strict)"("Value"=w185) -> ()  [unwired: 2 in, 2 out]
            n122 = property on="Scale Low Encoder Position" class="DigNum (strict)"("Value"=w184) -> ()  [unwired: 2 in, 2 out]
            n123 = property on="Scale Mid Encoder Position" class="DigNum (strict)"("Value"=w172) -> ()  [unwired: 2 in, 2 out]
            n124 = property on="Portal Encoder Position" class="DigNum (strict)"("Value"=w152) -> ()  [unwired: 2 in, 2 out]
            n125 = property on="Turn Distance P" class="DigNum (strict)"("Value"=w200) -> ()  [unwired: 2 in, 2 out]
            n126 = property on="Turn Distance I" class="DigNum (strict)"("Value"=w199) -> ()  [unwired: 2 in, 2 out]
            n127 = property on="Turn Distance D" class="DigNum (strict)"("Value"=w198) -> ()  [unwired: 2 in, 2 out]
            n128 = property on="Kp Upper" class="DigNum (strict)"("Value"=w197) -> ()  [unwired: 2 in, 2 out]
            n129 = property on="Ki Upper" class="DigNum (strict)"("Value"=w196) -> ()  [unwired: 2 in, 2 out]
            n130 = property on="Kd Upper" class="DigNum (strict)"("Value"=w195) -> ()  [unwired: 2 in, 2 out]
            n131 = property on="Kp Lower" class="DigNum (strict)"("Value"=w178) -> ()  [unwired: 2 in, 2 out]
            n132 = property on="Ki Lower" class="DigNum (strict)"("Value"=w177) -> ()  [unwired: 2 in, 2 out]
            n133 = property on="Kd Lower" class="DigNum (strict)"("Value"=w176) -> ()  [unwired: 2 in, 2 out]
            n134 = property on="Cube P" class="DigNum (strict)"("Value"=w179) -> ()  [unwired: 2 in, 2 out]
            n135 = property on="Cube I" class="DigNum (strict)"("Value"=w180) -> ()  [unwired: 2 in, 2 out]
            n136 = property on="Cube D" class="DigNum (strict)"("Value"=w181) -> ()  [unwired: 2 in, 2 out]
            n137 = property on="Number of Loops to be in Acceptable Error" class="DigNum (strict)"("Value"=w175) -> ()  [unwired: 2 in, 2 out]
            n138 = property on="Number of Loops to be in Tolerance" class="DigNum (strict)"("Value"=w174) -> ()  [unwired: 2 in, 2 out]
            n139 = property on="Turning Acceptable Tolerance" class="DigNum (strict)"("Value"=w173) -> ()  [unwired: 2 in, 2 out]
            n140 = property on="Turning Acceptable Error" class="DigNum (strict)"("Value"=w162) -> ()  [unwired: 2 in, 2 out]
            n141 = property on="Cube PID Acceptable Error" class="DigNum (strict)"("Value"=w161) -> ()  [unwired: 2 in, 2 out]
            n142 = property on="Left Low Gear P" class="DigNum (strict)"("Value"=w213) -> ()  [unwired: 2 in, 2 out]
            n143 = property on="Left Low Gear I" class="DigNum (strict)"("Value"=w212) -> ()  [unwired: 2 in, 2 out]
            n144 = property on="Left Low Gear D" class="DigNum (strict)"("Value"=w211) -> ()  [unwired: 2 in, 2 out]
            n145 = property on="Left Low Gear F" class="DigNum (strict)"("Value"=w210) -> ()  [unwired: 2 in, 2 out]
            n146 = property on="Left High Gear P" class="DigNum (strict)"("Value"=w209) -> ()  [unwired: 2 in, 2 out]
            n147 = property on="Left High Gear I" class="DigNum (strict)"("Value"=w208) -> ()  [unwired: 2 in, 2 out]
            n148 = property on="Left High Gear D" class="DigNum (strict)"("Value"=w207) -> ()  [unwired: 2 in, 2 out]
            n149 = property on="Left High Gear F" class="DigNum (strict)"("Value"=w206) -> ()  [unwired: 2 in, 2 out]
            n150 = property on="Right Low Gear P" class="DigNum (strict)"("Value"=w160) -> ()  [unwired: 2 in, 2 out]
            n151 = property on="Right Low Gear I" class="DigNum (strict)"("Value"=w159) -> ()  [unwired: 2 in, 2 out]
            n152 = property on="Right Low Gear D" class="DigNum (strict)"("Value"=w158) -> ()  [unwired: 2 in, 2 out]
            n153 = property on="Right Low Gear F" class="DigNum (strict)"("Value"=w157) -> ()  [unwired: 2 in, 2 out]
            n154 = property on="Right High Gear P" class="DigNum (strict)"("Value"=w156) -> ()  [unwired: 2 in, 2 out]
            n155 = property on="Right High Gear I" class="DigNum (strict)"("Value"=w155) -> ()  [unwired: 2 in, 2 out]
            n156 = property on="Right High Gear D" class="DigNum (strict)"("Value"=w154) -> ()  [unwired: 2 in, 2 out]
            n157 = property on="Right High Gear F" class="DigNum (strict)"("Value"=w153) -> ()  [unwired: 2 in, 2 out]
            n158 = Equal To 0?(x=w164) -> (x = 0?=w163:bool)
            n159 = call-poly <vilib>:"NT Write Value.vi"("Boolean"=w163, "Name"="Read?") -> ()  [unwired: 9 in, 1 out]
          }
          frame "Write" {
            # "Auto"
            # "RPED"
            # "Lift"
            # "Intake Rotation"
            # "Drive"
            n160 = Build Array("Left Forward Power", "Right Forward Power", "Left Backward Power", "Right Backward Power") -> (w317:dbl[])
            n161 = Build Array("Intake Rot Stow Encoder Position", "Intake Rot Scale High Encoder Position", "Intake Rot Scale Mid Encoder Position", "Intake Rot Scale Low Encoder Position", "Intake Rot Load Encoder Position", "Intake Rot Manual Up Power", "Intake Rot Manual Down Power", "Intake Rot Climb Encoder Positon", "Intake Rot Switch Encoder Position", "Intake Rot Exchange Encoder Position", "Intake Rot Portal Encoder Position") -> (w316:dbl[])
            n162 = Array To Spreadsheet String(array=w317, 3:"%f" ("format string")) -> (spreadsheet string=w300:string)  [unwired: 1 in]
            n163 = Build Array("Turn Distance P", "Turn Distance I", "Turn Distance D", "Kp Upper", "Ki Upper", "Kd Upper", "Kp Lower", "Ki Lower", "Kd Lower", "Cube P", "Cube I", "Cube D", "Number of Loops to be in Acceptable Error", "Number of Loops to be in Tolerance", "Turning Acceptable Tolerance", "Turning Acceptable Error", "Cube PID Acceptable Error") -> (w276:dbl[])
            n164 = Build Array("Left Low Gear P", "Left Low Gear I", "Left Low Gear D", "Left Low Gear F", "Left High Gear P", "Left High Gear I", "Left High Gear D", "Left High Gear F", "Right Low Gear P", "Right Low Gear I", "Right Low Gear D", "Right  Low Gear F", "Right High Gear P", "Right High Gear I", "Right High Gear D", "Right High Gear F") -> (w292:dbl[])
            n165 = Array To Spreadsheet String(array=w316, 3:"%f" ("format string")) -> (spreadsheet string=w303:string)  [unwired: 1 in]
            n166 = Build Array("Manual Up Power", "Manual Down Power", "Scale High Encoder Position", "Scale Low Encoder Position", "Scale Mid Encoder Position", "Switch Encoder Position", "Stow Encoder Position", "Climb Encoder Position", "Load Encoder Position", "Exchange Encoder Position", "Climb Power", "Portal Encoder Position") -> (w315:dbl[])
            n167 = call-poly <vilib>:"NT Write Value.vi"("String"=w300, "Name"="RPED Cals") -> ()  [unwired: 9 in, 1 out]
            n168 = Array To Spreadsheet String(array=w276, 3:"%f" ("format string")) -> (spreadsheet string=w285:string)  [unwired: 1 in]
            n169 = Array To Spreadsheet String(array=w292, 3:"%f" ("format string")) -> (spreadsheet string=w295:string)  [unwired: 1 in]
            n170 = Array To Spreadsheet String(array=w315, 3:"%f" ("format string")) -> (spreadsheet string=w302:string)  [unwired: 1 in]
            n171 = call-poly <vilib>:"NT Write Value.vi"("String"=w303, "Name"="Intake Rotation Cals") -> ()  [unwired: 9 in, 1 out]
            n172 = call-poly <vilib>:"NT Write Value.vi"("String"=w285, "Name"="Auto Cals") -> ()  [unwired: 9 in, 1 out]
            n173 = call-poly <vilib>:"NT Write Value.vi"("String"=w295, "Name"="Drive Cals") -> ()  [unwired: 9 in, 1 out]
            n174 = call-poly <vilib>:"NT Write Value.vi"("String"=w302, "Name"="Lift Cals") -> ()  [unwired: 9 in, 1 out]
          }
          frame "Show" {
            # "Auto"
            # "RPED SS"
            # "Lift SS"
            # "Rotation SS"
            # "Drive SS"
            n175 = local read "Number of Loops to be in Acceptable Error"() -> (→"Current Number of Loops to be in Acceptable Error":dbl)
            n176 = local read "Number of Loops to be in Tolerance"() -> (→"Current Number of Loops to be in Tolerance":dbl)
            n177 = local read "Intake Rot Scale High Encoder Position"() -> (→"Current Intake Rot Scale High Encoder Position":dbl)
            n178 = local read "Intake Rot Scale Low Encoder Position"() -> (→"Current Intake Rot Scale Low Encoder Position":dbl)
            n179 = local read "Intake Rot Scale Mid Encoder Position"() -> (→"Current Intake Rot Scale Mid Encoder Position":dbl)
            n180 = local read "Intake Rot Exchange Encoder Position"() -> (→"Current Intake Rot Exchange Encoder Position":dbl)
            n181 = local read "Intake Rot Portal Encoder Position"() -> (→"Current Intake Rot Portal Encoder Position":dbl)
            n182 = local read "Turning Acceptable Tolerance"() -> (→"Current Turning Acceptable Tolerance":dbl)
            n183 = local read "Intake Rot Switch Encoder Position"() -> (→"Current Intake Rot Switch Encoder Position":dbl)
            n184 = local read "Scale High Encoder Position"() -> (→"Current Scale High Encoder Position":dbl)
            n185 = local read "Intake Rot Climb Encoder Positon"() -> (→"Current Intake Rot Climb Encoder Position":dbl)
            n186 = local read "Intake Rot Stow Encoder Position"() -> (→"Current Intake Rot Stow Encoder Position":dbl)
            n187 = local read "Intake Rot Load Encoder Position"() -> (→"Current Intake Rot Load Encoder Position":dbl)
            n188 = local read "Scale Low Encoder Position"() -> (→"Current Scale Low Encoder Position":dbl)
            n189 = local read "Scale Mid Encoder Position"() -> (→"Current Scale Mid Encoder Position":dbl)
            n190 = local read "Exchange Encoder Position"() -> (→"Current Exchange Encoder Position":dbl)
            n191 = local read "Intake Rot Manual Down Power"() -> (→"Current Intake Rot Manual Down Power":dbl)
            n192 = local read "Switch Encoder Position"() -> (→"Current Switch Encoder Position":dbl)
            n193 = local read "Cube PID Acceptable Error"() -> (→"Current Cube PID Acceptable Error":dbl)
            n194 = local read "Climb Encoder Position"() -> (→"Current Climb Encoder Position":dbl)
            n195 = local read "Intake Rot Manual Up Power"() -> (→"Current Intake Rot Manual Up Power":dbl)
            n196 = local read "Turning Acceptable Error"() -> (→"Current Turning Acceptable Error":dbl)
            n197 = local read "Stow Encoder Position"() -> (→"Current Stow Encoder Position":dbl)
            n198 = local read "Load Encoder Position"() -> (→"Current Load Encoder Position":dbl)
            n199 = local read "Portal Encoder Position"() -> (→"Current Portal Encoder Position":dbl)
            n200 = local read "Manual Down Power"() -> (→"Current Manual Down Power":dbl)
            n201 = local read "Right Backward Power"() -> (→"Current Right Backward Power":dbl)
            n202 = local read "Manual Up Power"() -> (→"Current Manual Up Power":dbl)
            n203 = local read "Right Forward Power"() -> (→"Current Right Forward Power":dbl)
            n204 = local read "Left Backward Power"() -> (→"Current Left Backward Power":dbl)
            n205 = local read "Left Forward Power"() -> (→"Current Left Forward Power":dbl)
            n206 = local read "Turn Distance D"() -> (→"Current Turn Distance D":dbl)
            n207 = local read "Turn Distance P"() -> (→"Current Turn Distance P":dbl)
            n208 = local read "Turn Distance I"() -> (→"Current Turn Distance I":dbl)
            n209 = local read "Climb Power"() -> (→"Current Climb Power":dbl)
            n210 = local read "Left Low Gear P"() -> (→"Current Left Low Gear P":dbl)
            n211 = local read "Left High Gear P"() -> (→"Current Left High Gear P":dbl)
            n212 = local read "Left Low Gear I"() -> (→"Current Left Low Gear I":dbl)
            n213 = local read "Left High Gear I"() -> (→"Current Left High Gear I":dbl)
            n214 = local read "Kp Upper"() -> (→"Current Kp Upper":dbl)
            n215 = local read "Kd Upper"() -> (→"Current Kd Upper":dbl)
            n216 = local read "Kp Lower"() -> (→"Current Kp Lower":dbl)
            n217 = local read "Kd Lower"() -> (→"Current Kd Lower":dbl)
            n218 = local read "Right High Gear F"() -> (→"Current Right High Gear F":dbl)
            n219 = local read "Ki Upper"() -> (→"Current Ki Upper":dbl)
            n220 = local read "Ki Lower"() -> (→"Current Ki Lower":dbl)
            n221 = local read "Right  Low Gear F"() -> (→"Current Right Low Gear F":dbl)
            n222 = local read "Right High Gear D"() -> (→"Current Right High Gear D":dbl)
            n223 = local read "Right High Gear I"() -> (→"Current Right High Gear I":dbl)
            n224 = local read "Right High Gear P"() -> (→"Current Right High Gear P":dbl)
            n225 = local read "Right Low Gear I"() -> (→"Current Right Low Gear I":dbl)
            n226 = local read "Right Low Gear P"() -> (→"Current Right Low Gear P":dbl)
            n227 = local read "Right Low Gear D"() -> (→"Current Right Low Gear D":dbl)
            n228 = local read "Cube D"() -> (→"Current Cube D":dbl)
            n229 = local read "Cube P"() -> (→"Current Cube P":dbl)
            n230 = local read "Left Low Gear D"() -> (→"Current Left Low Gear D":dbl)
            n231 = local read "Left High Gear F"() -> (→"Current Left High Gear F":dbl)
            n232 = local read "Left Low Gear F"() -> (→"Current Left Low Gear F":dbl)
            n233 = local read "Cube I"() -> (→"Current Cube I":dbl)
            n234 = local read "Left High Gear D"() -> (→"Current Left High Gear D":dbl)
          }
        }
        "Drive" <- w141
        "Intake Rotation" <- w141
        "RPED" <- w141
        "Lift" <- w141
        "Auto" <- w141
      }
    }
  }
  n235 = Bundle("Camera Image"=w51, "Dashboard Tab"=w50, "Background"=w46, "Rec Mode"=w39, "Test Slider"=w38, "On/Off"=w37, "Test Ring"=w36, "Rev/Fwd"=w35, "Test Name"=w41, "Motor"=w40, "Progress"=w34, "CheckList"=w44, "Tree"=w43, "Test Tree"=w42, "Command Params"=w29, "Command Selection"=w26, "Execute Command"=w28, "Cmd Status"=w22, "Camera Settings"=w18, "Camera Name"=w17, "Camera Info"=w16, "Camera Settings Right"=w8, "Camera Name Right"=w7, "Camera Image Right"=w6) -> (w45:T17)  [unwired: 1 in]
  n236 = call "Handle Camera Configuration.vi"("CameraNameRef"=w19, "Display Name"=w1, "ClusterRef"=w20) -> ()  [unwired: 9 in]
  n237 = disable-structure shown="Disabled" {
    disable-tunnel: w55 -> [w384 _]
    disable-tunnel: w47 -> [w383 _]
    disable-tunnel: w45 -> [w382 _]
    disable-tunnel: w31 -> [w381 _]
    frame Disabled {
      n238 = call "Adjust Dashboard Window.vi"("Sizing Refnums"=w382, "Size Constraints"=w383, "VI"=w384, "WIn Mode"=w381) -> ()  [unwired: 8 in]
    }
    frame Enabled {
    }
  }
  n239 = call "Handle Camera Configuration.vi"("CameraNameRef"=w9, "Display Name"=w2, "ClusterRef"=w10) -> ()  [unwired: 9 in]
  n240 = register-events(refnum<vi> refnum, w23) -> (reference out=w60:refnum<event-registration>, error out=w59:errorcluster)  [unwired: 2 in]
  n241 = call "Initialize Camera and CheckList.vi"("ListBox in"=w44) -> ()  [unwired: 11 in]
  n242 = vi-ref "Playback Controls.vi"() -> (w61:refnum<vi>)
  n243 = property class="VI"() -> ("Panel"=w63:refnum<vi>)  [unwired: 2 in, 2 out]
  n244 = while {
    tunnel: w52 -> [w396]
    tunnel: w32 -> [w394]
    tunnel: [w392] -> _
    tunnel: u32 1000 ("milliseconds to wait") -> [w391]
    tunnel: w23 -> [w385]
    i -> [w392]
    stop <- FALSE stop-if-true
    n245 = local read "Rec Mode"() -> (w387:enum32{"Stop", "Record", "Playback"})
    n246 = Wait on Notification(notifier=w394, timeout in ms (-1)=w391) -> (notification=w393:string, timed out?=w389:bool)  [unwired: 2 in, 2 out]
    n247 = Equal?(x=w387, y=u16 2 ("Rec Mode")) -> (x = y?=w388:bool)
    n248 = Compound Arithmetic op=OR(invert w389, w388) -> (w390:bool)
    n249 = case shown="True" w390 {
      tunnel: w396 -> [_ w399]
      tunnel: w393 -> [_ w398]
      tunnel: w385 -> [_ w397]
      frame False {
      }
      frame True {
        n250 = call <vilib>:"Bind Controls to SmartDashboard.vi"("RPC ref"=w397, "Bound Control Refs"=w399, "Server IP Address"=w398) -> ()  [unwired: 9 in]
      }
    }
  }
  n251 = property class="Pnl"(reference=w63) -> ("Panes[]"=w64:refnum<vi>[])  [unwired: 1 in, 2 out]
  n252 = while {
    tunnel: w12 -> [w414]
    tunnel: w11 -> [_]
    tunnel: [w409] -> _
    tunnel: w3 -> [w403]
    tunnel: w2 -> [w400]
    i -> [w409]
    stop <- FALSE stop-if-true
    n253 = local read "NT Connection"() -> (w404:bool)
    n254 = local read "Rec Mode"() -> (w413:enum32{"Stop", "Record", "Playback"})
    n255 = Bundle("Camera Name Right"="Camera Name Right", w400, "Saved DB Images Info"=w403) -> (w402:T18)  [unwired: 1 in]
    n256 = call <vilib>:"WPI_CameraRead MJPG for Dashboard.vi"("Camera Settings"="Camera Settings Right", "Rec Mode"=w413, "NT Connection"=w404, "Capture Info"=w402, "Refnum in"=w414) -> ("Active"=w408:bool, "Refnum out"=w411:T1, "FPS"=w406:dbl, "Bandwidth (Mbps)"=w407:dbl)  [unwired: 3 in]
    n257 = case shown="False" w408 {
      tunnel: w411 -> [w415 w417]
      tunnel: w407 -> [_ _]
      tunnel: w406 -> [_ _]
      tunnel: [w415 w417] -> w405
      frame False {
        n258 = Wait Until Next ms Multiple(millisecond multiple=u32 500) -> ()  [unwired: 1 out]
      }
      frame True {
      }
    }
    "Camera Image Right" <- w405
  }
  n259 = Index Array(array=w64) -> (element=w62:refnum<vi>)  [unwired: 1 in]
  n260 = control-ref of="Test Tree"() -> (w65:refnum<vi>)
  n261 = while {
    tunnel: w71 -> [w430]
    tunnel: w70 -> [_]
    tunnel: [w431] -> _
    tunnel: w3 -> [w421]
    tunnel: w1 -> [w418]
    i -> [w431]
    stop <- FALSE stop-if-true
    # "Optionally read the DB image,\nlog, or retrieve images from a\nlogged match"
    n262 = local read "NT Connection"() -> (w422:bool)
    n263 = local read "Rec Mode"() -> (w426:enum32{"Stop", "Record", "Playback"})
    n264 = Bundle("Camera Name"="Camera Name", w418, "Saved DB Images Info"=w421) -> (w420:T19)  [unwired: 1 in]
    n265 = call <vilib>:"WPI_CameraRead MJPG for Dashboard.vi"("Camera Settings"="Camera Settings", "Rec Mode"=w426, "NT Connection"=w422, "Capture Info"=w420, "Refnum in"=w430) -> ("Active"=w428:bool, "Refnum out"=w429:T1, "FPS"=w427:dbl, "Bandwidth (Mbps)"=w425:dbl)  [unwired: 3 in]
    n266 = case shown="True" w428 {
      tunnel: w429 -> [w433 w444]
      tunnel: w425 -> [_ w441]
      tunnel: w427 -> [_ w442]
      tunnel: [w433 w438] -> w423
      frame False {
        w435 = u32 1985280 ("Color Box")
        # "Sleep for 500ms"
        n267 = Bundle("Color Box"=w435, "Color Box"=w435) -> (w436:cluster{"Color Box":u32, "Color Box":u32})  [unwired: 1 out]
        n268 = Build Array(w436) -> (w434:cluster{"Color Box":u32, "Color Box":u32}[])
        n269 = property on="Mbps LED" class="Bool (strict)"("Colors [4]"=w434) -> ()  [unwired: 2 in, 2 out]
        n270 = Wait Until Next ms Multiple(millisecond multiple=u32 500) -> ()  [unwired: 1 out]
      }
      frame True {
        # "Here is where you would annotate,\npossibly process, and display the image"
        # "Update Mbps LED"
        n271 = case shown="Default" w441 {
          tunnel: [u32 6618880 ("Color Box") u32 16776722 ("Color Box") u32 16716800 ("Color Box")] -> w445
          frame Default {
          }
          frame 4, 5 {
          }
          frame 6.. {
          }
        }
        n272 = call "IMAQ Clear Overlay"("Image"=w444) -> ("error out"=w447:errorcluster, "Image Out"=w438:T1)  [unwired: 2 in, 7 out]
        n273 = Bundle(FALSE, "Bandwidth (Mbps)"=w441, "FPS"=w442) -> (→"Camera Info":cluster{bool, "Bandwidth (Mbps)":dbl, "FPS":dbl})  [unwired: 1 in]
        n274 = Bundle("Color Box"=w445, "Color Box"=w445) -> (w446:cluster{"Color Box":u32, "Color Box":u32})  [unwired: 1 out]
        n275 = Unbundle By Name(w447) -> ("status"=w448:bool)
        n276 = Build Array(w446) -> (w443:cluster{"Color Box":u32, "Color Box":u32}[])
        n277 = property on="Image Message" class="Str"("Visible"=w448) -> ()  [unwired: 2 in, 2 out]
        n278 = property on="Mbps LED" class="Bool (strict)"("Colors [4]"=w443) -> ()  [unwired: 2 in, 2 out]
      }
    }
    "Camera Image" <- w423
  }
  n279 = while {
    tunnel: [w461] -> _
    tunnel: w65 -> [w460]
    tunnel: w61 -> [w459]
    tunnel: w60 -> [w458]
    tunnel: w59 -> [_]
    tunnel: w55 -> [w457]
    tunnel: w23 -> [w456]
    tunnel: w21 -> [w455]
    shift-right: [w454] -> _
    shift-left: _ -> [w453]
    tunnel: w15 -> [w452]
    i -> [w461]
    stop <- FALSE stop-if-true
    n280 = event shown="[0] Timeout" {
      selector: w458 -> [_ _ _ _ _ _ _ _ _ _ _ _ _ _ _ _ _ _ _]
      dyn-events: [_ _ _ _ _ _ _ _ _ _ _ _ _ _ w715 _ _ _ _] -> _
      timeout: u32 60 ("milliseconds to wait") -> [_ _ _ _ _ _ _ _ _ _ _ _ _ _ _ _ _ _ _]
      tunnel: w460 -> [w473 _ _ _ _ _ _ _ _ _ _ _ _ _ _ _ _ _ _]
      tunnel: "Test Tree" -> [_ _ _ _ _ _ _ _ _ w682 w690 w692 w696 w704 _ _ _ _ _]
      tunnel: w459 -> [_ _ _ _ _ _ _ _ _ _ _ _ _ _ w717 _ w735 _ _]
      tunnel: w457 -> [_ _ _ _ _ _ _ _ _ _ _ _ _ _ w713 _ _ _ _]
      tunnel: w456 -> [_ _ _ _ _ _ _ _ _ _ _ _ _ _ w711 _ _ _ _]
      tunnel: w455 -> [w468 _ _ _ w633 _ _ _ _ _ _ _ _ _ _ _ _ _ _]
      tunnel: [w467 w516 w618 w623 w631 w640 w650 w657 w669 w681 w688 w691 w695 w703 w710 w730 w732 w736 w749] -> w454
      tunnel: w453 -> [w467 w516 w618 w623 w631 _ _ w657 w669 w681 w688 w691 w695 w703 w710 w730 w732 w736 w749]
      tunnel: w452 -> [w465 _ _ _ _ _ _ _ _ _ _ _ _ _ _ _ _ _ _]
      event Timeout {
        n281 = event-data() -> ()  [unwired: 1 in, 1 out]
        n282 = local read "Mode"() -> (w470:T4)
        n283 = case shown="\"Basic\"" "Dashboard Tab" {
          tunnel: w473 -> [_ _ w489 _ _ _]
          tunnel: "TestMode/Automatic/" ("Name Pattern") -> [_ _ w488 _ _ _]
          tunnel: T20 [{"Operation"=enum."Clear", "Color Box"=14013909}, {"Operation"=enum."Clear", "Color Box"=14013909}, {"Operation"=enum."Clear", "Color Box"=14013909}, {"Operation"=enum."Clear", "Color Box"=14013909}, {"Operation"=enum."Update", "Color Box"=14013909}, {"Operation"=enum."Update", "Color Box"=16777215}, {"Operation"=enum."Clear", "Color Box"=14013909}, {"Operation"=enum."Clear", "Color Box"=14013909}, {"Operation"=enum."Clear", "Color Box"=14013909}] -> [_ _ w481 _ w509 _]
          tunnel: w470 -> [_ _ w480 _ w508 _]
          tunnel: u32[] [15790320, 15790320, 15790320, 15790320, 16777215, 16777215, 15790320, 15790320, 15790320] -> [_ _ _ _ w514 _]
          tunnel: w468 -> [_ _ _ _ w502 _]
          tunnel: w465 -> [_ w475 _ _ _ _]
          frame "Custom", Default {
          }
          frame "Basic" {
            n284 = call <vilib>:"WPI_DashboardUpdateNames.vi"("Controls on Tab"=w475) -> ()  [unwired: 11 in]
          }
          frame "Test" {
            w487 = -2 ("Active Item:Row Number")
            n285 = Index Array(array=w481, index=w480) -> (element=w482:T23)
            n286 = Unbundle(w482) -> ("Operation"=w483:enum16{"Update", "Clear"}, "Color Box"=w484:u32)
            n287 = call <vilib>:"NT Read String.vi"("Name"="TestMode/TestName") -> ("String"=w478:string)  [unwired: 9 in, 1 out]
            n288 = call <vilib>:"NT Read and Format Entries as Tree.vi"("Operation"=w483, "Name Pattern"=w488, "Tree Refnum"=w489) -> ()  [unwired: 7 in, 2 out]
            n289 = case shown="\"\"" w478 {
              tunnel: "TestMode/TestProgress" ("Name") -> [w491 _]
              tunnel: "TestMode/TestProgressText" ("Name") -> [w490 _]
              frame Default {
                n290 = call <vilib>:"NT Read Number.vi"("Name"=w491) -> ("Numeric"=w492:dbl)  [unwired: 9 in, 1 out]
                n291 = call <vilib>:"NT Read String.vi"("Name"=w490) -> ("String"=w493:string)  [unwired: 9 in, 1 out]
                n292 = Bundle("Numeric"=w492, "String"=w493) -> (→"Progress":cluster{"Numeric":dbl, "String":string})  [unwired: 1 in]
              }
              frame "" {
                n293 = property on="Progress" class="Clust (strict)"("Visible"=FALSE) -> ()  [unwired: 2 in, 2 out]
                n294 = local write "Test Name"(u16 0) -> ()
              }
            }
            n295 = property on="Test Tree" class="Tree (strict)"("Active Item Row Number"=w487, "ActiveColNum"=w487, "CellBG"=w484, "Active Item Row Number"=-1 ("Active Item:Row Number"), "CellBG"=u32 5789784 ("Color Box")) -> ()  [unwired: 2 in, 2 out]
          }
          frame "Variables" {
            w499 = string[] ["CameraPublisher", "Usage", "DB"]  # Items to initially close
            n296 = First Call?() -> (First Call?: T/F=w500:bool)
            n297 = control-ref of="Tree"() -> (w501:refnum<vi>)
            n298 = Select(t=w499, s=w500, f=string[] []) -> (s? t:f=w497:string[])
            n299 = call <vilib>:"NT Read and Format Entries as Tree.vi"("Tags to  Close"=w497, "Tree Refnum"=w501) -> ()  [unwired: 8 in, 2 out]
          }
          frame "Commands" {
            w510 = u32 5789784 ("Color Box")
            w511 = T24 {"Row"=-1, "Column"=-2} ("Active Cell:Active Cell")
            w513 = T24 {"Row"=-2, "Column"=-2} ("Active Cell:Active Cell")
            n300 = Index Array(array=w514, index=w508) -> (element=w512:u32)
            n301 = Index Array(array=w509, index=w508) -> (element=w507:T23)
            n302 = Unbundle(w507) -> ("Operation"=w506:enum16{"Update", "Clear"})  [unwired: 1 out]
            n303 = local read "Command Selection"() -> (w505:i32)
            n304 = property on="Command Selection" class="MCListbox (strict)"("ActiveCell"=w513, "CellBG"=w512, "ActiveCell"=w511, "CellBG"=w510) -> ()  [unwired: 2 in, 2 out]
            n305 = call <vilib>:"WPI_DashboardUpdate RPC Info.vi"("Operation"=w506) -> ("update"=w504:bool, "commands"=w503:string[][])  [unwired: 9 in]
            n306 = property on="Command Selection" class="MCListbox (strict)"("ItemNames"=w503) -> ()  [unwired: 2 in, 2 out]
            n307 = property on="Command Params" class="Tbl (strict)"("Active Cell"=w513, "Cell BG Color"=w512, "Active Cell"=w511, "Cell BG Color"=w510) -> ()  [unwired: 2 in, 2 out]
            n308 = call <vilib>:"WPI_DashboardUpdate Command Params.vi"("Update"=w504, "NewVal"=w505, "Commands"=w503, "Param Tbl"=w502) -> ()  [unwired: 7 in, 1 out]
          }
          frame "Checklist" {
          }
        }
        n309 = call <vilib>:"Connextion Info.vi"() -> ("Connected"=→"NT Connection":bool)  [unwired: 10 in, 1 out]
      }
      event "Test Tree": Value Change {
        # "Show appropriate\ncontrols"
        n310 = event-data() -> ("CtlRef"=w519:refnum<vi>, "NewVal"=w517:string)  [unwired: 1 in]
        n311 = call <vilib>:"WPI_UtilitiesGetTreeIOName.vi"("NewVal"=w517, "TreeControl in"=w519) -> ("I/O Name"=w520:string)  [unwired: 9 in]
        n312 = case shown="\"Camera\"" w520 {
          selector: w520 -> [_ w527 _ w549 w558 _]
          tunnel: w517 -> [_ _ w546 w548 _ w565]
          tunnel: cluster{string[]}[] [{["640x480", "320x240", "160x120"]}, {["Auto", "Fixed indoor", "Fixed outdoor 1", "Fixed outdoor 2", "Fixed fluorescent 1", "Fixed fluorescent 2", "Hold current"]}, {["Auto", "Flicker-free 50 Hz", "Flicker-free 60 Hz", "Hold current"]}, {["None", "Prioritize frame rate", "Prioritize image quality"]}, {["Monochrome", "Color"]}] -> [_ _ _ _ _ w564]
          frame Default {
            w522 = FALSE ("Visible")
            w521 = FALSE ("Visible")
            n313 = property on="Motor" class="Clust (strict)"("Visible"=w521) -> ()  [unwired: 2 in, 2 out]
            n314 = property on="Test Ring" class="Ring (strict)"("Visible"=w521) -> ()  [unwired: 2 in, 2 out]
            n315 = property on="Rev/Fwd" class="Clust (strict)"("Visible"=w522) -> ()  [unwired: 2 in, 2 out]
            n316 = property on="On/Off" class="Bool (strict)"("Visible"=w522) -> ()  [unwired: 2 in, 2 out]
            n317 = property on="Test Slider" class="Slide (strict)"("Visible"=w522) -> ()  [unwired: 2 in, 2 out]
          }
          frame "Analog Out", "Motor", "PWM" {
            w528 = FALSE ("Visible")
            n318 = case shown="\"Analog Out\"" w527 {
              tunnel: [1.0 ("Value") -1.0 ("Value") 0.0 ("Value")] -> w526
              tunnel: [255.0 ("Value") 1.0 ("Value") 5.0 ("Value")] -> w525
              tunnel: [128.0 ("Value") 0.0 ("Value") 0.0 ("Value")] -> w524
              tunnel: [64.0 ("Value") 0.5 ("Value") 1.0 ("Value")] -> w523
              frame "PWM" {
              }
              frame "Motor", Default {
              }
              frame "Analog Out" {
              }
            }
            n319 = property on="Motor" class="Clust (strict)"("Visible"=TRUE) -> ()  [unwired: 2 in, 2 out]
            n320 = property on="Value" class="Slide (strict)"("Value"=w524, "Scale.Minimum"=w526, "Scale.Maximum"=w525, "Scale.Increment"=w523) -> ()  [unwired: 2 in, 2 out]
            n321 = property on="On/Off" class="Bool (strict)"("Visible"=w528) -> ()  [unwired: 2 in, 2 out]
            n322 = property on="Test Slider" class="Slide (strict)"("Visible"=w528) -> ()  [unwired: 2 in, 2 out]
            n323 = property on="Test Ring" class="Ring (strict)"("Visible"=w528) -> ()  [unwired: 2 in, 2 out]
            n324 = property on="Rev/Fwd" class="Clust (strict)"("Visible"=w528) -> ()  [unwired: 2 in, 2 out]
          }
          frame "Servo" {
            w544 = FALSE ("Visible")
            n325 = call <vilib>:"NT Read Number.vi"("Name"=w546) -> ("Numeric"=w545:dbl)  [unwired: 9 in, 1 out]
            n326 = property on="Test Slider" class="Slide (strict)"("Visible"=TRUE, "Scale.Maximum"=170.0 ("Scale.Range:Maximum")) -> ()  [unwired: 2 in, 2 out]
            n327 = local write "Test Slider"(w545) -> ()
            n328 = property on="Motor" class="Clust (strict)"("Visible"=w544) -> ()  [unwired: 2 in, 2 out]
            n329 = property on="Rev/Fwd" class="Clust (strict)"("Visible"=w544) -> ()  [unwired: 2 in, 2 out]
            n330 = property on="On/Off" class="Bool (strict)"("Visible"=w544) -> ()  [unwired: 2 in, 2 out]
            n331 = property on="Test Ring" class="Ring (strict)"("Visible"=w544) -> ()  [unwired: 2 in, 2 out]
          }
          frame "Relay", "Solenoid" {
            w547 = FALSE ("Visible")
            n332 = property on="Motor" class="Clust (strict)"("Visible"=w547) -> ()  [unwired: 2 in, 2 out]
            n333 = property on="Test Slider" class="Slide (strict)"("Visible"=w547) -> ()  [unwired: 2 in, 2 out]
            n334 = Search and Replace String(input string=w548, search string="/Value  **", replace string="/Direction") -> (result string=w554:string)  [unwired: 5 in, 3 out]
            n335 = property on="Test Ring" class="Ring (strict)"("Visible"=w547) -> ()  [unwired: 2 in, 2 out]
            n336 = call <vilib>:"NT Read String.vi"("Name"=w554) -> ("String"=w552:string)  [unwired: 9 in, 1 out]
            n337 = Equal?(x="Both directions", y=w552) -> (x = y?=w550:bool)
            n338 = Not(x=w550) -> (.not. x?=w551:bool)
            n339 = property on="Rev/Fwd" class="Clust (strict)"("Visible"=w550) -> ()  [unwired: 2 in, 2 out]
            n340 = property on="On/Off" class="Bool (strict)"("Visible"=w551, "Caption.Text"=w549) -> ()  [unwired: 2 in, 2 out]
          }
          frame "Compressor", "Digital Out" {
            w557 = FALSE ("Visible")
            # "Get direction and finish"
            n341 = property on="Motor" class="Clust (strict)"("Visible"=w557) -> ()  [unwired: 2 in, 2 out]
            n342 = property on="Test Slider" class="Slide (strict)"("Visible"=w557) -> ()  [unwired: 2 in, 2 out]
            n343 = property on="Test Ring" class="Ring (strict)"("Visible"=w557) -> ()  [unwired: 2 in, 2 out]
            n344 = property on="On/Off" class="Bool (strict)"("Visible"=TRUE, "Caption.Text"=w558) -> ()  [unwired: 2 in, 2 out]
            n345 = property on="Rev/Fwd" class="Clust (strict)"("Visible"=FALSE) -> ()  [unwired: 2 in, 2 out]
          }
          frame "Camera" {
            n346 = call <vilib>:"Get Last Path Segment.vi"("String in"=w565) -> ("String out"=w566:string)  [unwired: 10 in]
            n347 = property on="On/Off" class="Bool (strict)"("Visible"=FALSE) -> ()  [unwired: 2 in, 2 out]
            n348 = property on="Motor" class="Clust (strict)"("Visible"=FALSE) -> ()  [unwired: 2 in, 2 out]
            n349 = property on="Rev/Fwd" class="Clust (strict)"("Visible"=FALSE) -> ()  [unwired: 2 in, 2 out]
            n350 = case shown="\"White Balance  **\"" w566 {
              tunnel: w565 -> [w572 w581 w590 w599 w608 _ w614]
              tunnel: w564 -> [w570 w578 w587 w596 w605 _ _]
              frame "Size  **" {
                n351 = Index Array(array=w570) -> (element=w569:cluster{string[]})  [unwired: 1 in]
                n352 = call <vilib>:"NT Read String.vi"("Name"=w572) -> ("String"=w571:string)  [unwired: 9 in, 1 out]
                n353 = Unbundle(w569) -> (w567:string[])
                n354 = Match First String(2:w567, 3:w571) -> (0:w568:i32)  [unwired: 1 out]
                n355 = property on="Test Ring" class="Ring (strict)"("Value"=w568, "Strings []"=w567) -> ()  [unwired: 2 in, 2 out]
                n356 = property on="Test Ring" class="Ring (strict)"("Visible"=TRUE) -> ()  [unwired: 2 in, 2 out]
                n357 = property on="Test Slider" class="Slide (strict)"("Visible"=FALSE) -> ()  [unwired: 2 in, 2 out]
              }
              frame "White Balance  **" {
                n358 = Index Array(array=w578, index=1) -> (element=w579:cluster{string[]})
                n359 = call <vilib>:"NT Read String.vi"("Name"=w581) -> ("String"=w580:string)  [unwired: 9 in, 1 out]
                n360 = Unbundle(w579) -> (w576:string[])
                n361 = Match First String(2:w576, 3:w580) -> (0:w575:i32)  [unwired: 1 out]
                n362 = property on="Test Ring" class="Ring (strict)"("Value"=w575, "Strings []"=w576) -> ()  [unwired: 2 in, 2 out]
                n363 = property on="Test Ring" class="Ring (strict)"("Visible"=TRUE) -> ()  [unwired: 2 in, 2 out]
                n364 = property on="Test Slider" class="Slide (strict)"("Visible"=FALSE) -> ()  [unwired: 2 in, 2 out]
              }
              frame "Exposure  **" {
                n365 = Index Array(array=w587, index=2) -> (element=w588:cluster{string[]})
                n366 = call <vilib>:"NT Read String.vi"("Name"=w590) -> ("String"=w589:string)  [unwired: 9 in, 1 out]
                n367 = Unbundle(w588) -> (w584:string[])
                n368 = Match First String(2:w584, 3:w589) -> (0:w585:i32)  [unwired: 1 out]
                n369 = property on="Test Ring" class="Ring (strict)"("Value"=w585, "Strings []"=w584) -> ()  [unwired: 2 in, 2 out]
                n370 = property on="Test Ring" class="Ring (strict)"("Visible"=TRUE) -> ()  [unwired: 2 in, 2 out]
                n371 = property on="Test Slider" class="Slide (strict)"("Visible"=FALSE) -> ()  [unwired: 2 in, 2 out]
              }
              frame "Exposure Priority  **" {
                n372 = Index Array(array=w596, index=3) -> (element=w597:cluster{string[]})
                n373 = call <vilib>:"NT Read String.vi"("Name"=w599) -> ("String"=w598:string)  [unwired: 9 in, 1 out]
                n374 = Unbundle(w597) -> (w593:string[])
                n375 = Match First String(2:w593, 3:w598) -> (0:w594:i32)  [unwired: 1 out]
                n376 = property on="Test Ring" class="Ring (strict)"("Value"=w594, "Strings []"=w593) -> ()  [unwired: 2 in, 2 out]
                n377 = property on="Test Ring" class="Ring (strict)"("Visible"=TRUE) -> ()  [unwired: 2 in, 2 out]
                n378 = property on="Test Slider" class="Slide (strict)"("Visible"=FALSE) -> ()  [unwired: 2 in, 2 out]
              }
              frame "Color Enable  **" {
                n379 = Index Array(array=w605, index=4) -> (element=w606:cluster{string[]})
                n380 = call <vilib>:"NT Read String.vi"("Name"=w608) -> ("String"=w607:string)  [unwired: 9 in, 1 out]
                n381 = Unbundle(w606) -> (w602:string[])
                n382 = Match First String(2:w602, 3:w607) -> (0:w603:i32)  [unwired: 1 out]
                n383 = property on="Test Ring" class="Ring (strict)"("Value"=w603, "Strings []"=w602) -> ()  [unwired: 2 in, 2 out]
                n384 = property on="Test Ring" class="Ring (strict)"("Visible"=TRUE) -> ()  [unwired: 2 in, 2 out]
                n385 = property on="Test Slider" class="Slide (strict)"("Visible"=FALSE) -> ()  [unwired: 2 in, 2 out]
              }
              frame Default {
                n386 = property on="Test Ring" class="Ring (strict)"("Visible"=FALSE) -> ()  [unwired: 2 in, 2 out]
                n387 = property on="Test Slider" class="Slide (strict)"("Visible"=FALSE) -> ()  [unwired: 2 in, 2 out]
              }
              frame "Brightness  **", "Color Level  **", "Compression  **", "FPS  **", "Sharpness  **" {
                n388 = call <vilib>:"NT Read Number.vi"("Name"=w614) -> ("Numeric"=w613:dbl)  [unwired: 9 in, 1 out]
                n389 = local write "Test Slider"(w613) -> ()
                n390 = property on="Test Slider" class="Slide (strict)"("Visible"=TRUE, "Scale.Maximum"=100.0 ("Scale.Range:Maximum")) -> ()  [unwired: 2 in, 2 out]
                n391 = property on="Test Ring" class="Ring (strict)"("Visible"=FALSE) -> ()  [unwired: 2 in, 2 out]
              }
            }
          }
        }
        n392 = property on="Progress" class="Clust (strict)"("Visible"=FALSE) -> ()  [unwired: 2 in, 2 out]
      }
      event "Test Name": Mouse Enter {
        # "Populate the ring with the list of tests"
        n393 = event-data() -> ()  [unwired: 1 in, 1 out]
        n394 = call <vilib>:"NT Read String Array.vi"("Name"="TestMode/TestList") -> ("String Array"=w622:string[])  [unwired: 9 in, 1 out]
        n395 = Build Array (concatenate)("Select the test to run...", w622) -> (w621:string[])
        n396 = property on="Test Name" class="Ring (strict)"("Strings []"=w621) -> ()  [unwired: 2 in, 2 out]
      }
      event "Test Name": Value Change {
        w624 = FALSE ("Visible")
        # "Tell the robot the test name to run"
        n397 = event-data() -> ("NewVal"=w628:u16)  [unwired: 1 in]
        n398 = property on="Test Name" class="Ring (strict)"() -> ("Strings []"=w629:string[])  [unwired: 2 in, 2 out]
        n399 = local write "Progress"(T8 {"Test Progress"=0, "Test Progress Text"=""} ("Progress")) -> ()
        n400 = Index Array(array=w629, index=w628) -> (element=w627:string)
        n401 = call <vilib>:"NT Write String.vi"("String"=w627, "Name"="TestMode/TestName") -> ()  [unwired: 9 in, 1 out]
        n402 = property on="Progress" class="Clust (strict)"("Visible"=TRUE) -> ()  [unwired: 2 in, 2 out]
        n403 = property on="Motor" class="Clust (strict)"("Visible"=w624) -> ()  [unwired: 2 in, 2 out]
        n404 = property on="Test Slider" class="Slide (strict)"("Visible"=w624) -> ()  [unwired: 2 in, 2 out]
        n405 = property on="On/Off" class="Bool (strict)"("Visible"=w624) -> ()  [unwired: 2 in, 2 out]
        n406 = property on="Rev/Fwd" class="Clust (strict)"("Visible"=w624) -> ()  [unwired: 2 in, 2 out]
        n407 = property on="Test Ring" class="Ring (strict)"("Visible"=w624) -> ()  [unwired: 2 in, 2 out]
      }
      event "Command Selection": Value Change {
        # "Get the params and show in table"
        n408 = event-data() -> ("NewVal"=w634:i32)  [unwired: 1 in]
        n409 = property on="Command Selection" class="MCListbox (strict)"() -> ("ItemNames"=w632:string[][])  [unwired: 2 in, 2 out]
        n410 = call <vilib>:"WPI_DashboardUpdate Command Params.vi"("NewVal"=w634, "Commands"=w632, "Param Tbl"=w633) -> ()  [unwired: 8 in, 1 out]
      }
      event "Execute Command": Value Change {
        # "Started one, Unique ID holds\nresponse"
        n411 = event-data() -> ()  [unwired: 1 in, 1 out]
        n412 = property on="Command Selection" class="MCListbox (strict)"() -> ("ItemNames"=w645:string[][])  [unwired: 2 in, 2 out]
        n413 = Index Array(array=w645, index (row)="Command Selection", index (col)=0) -> (element=w643:string)
        n414 = call <vilib>:"Invoke Commands.vi"("Command Params"="Command Params", "Function Name"=w643) -> ("Params"=w639:u8, "Started"=w638:bool)  [unwired: 7 in, 1 out]
        n415 = Array Subset(array="Command Params", length (row)=w639) -> (w640:string[][])  [unwired: 3 in]
        n416 = Select(t="Executing" ("Cmd Status"), s=w638, f="" ("Cmd Status")) -> (s? t:f=→"Cmd Status":string)
      }
      event "Command Selection": Double Click {
        n417 = event-data() -> ("Row"=w653:i32)  [unwired: 1 in]
        n418 = property on="Command Selection" class="MCListbox (strict)"() -> ("ItemNames"=w656:string[][])  [unwired: 2 in, 2 out]
        n419 = local read "Command Params"() -> (w652:string[][])
        n420 = Index Array(array=w656, index (row)=w653, index (col)=0) -> (element=w654:string)
        n421 = call <vilib>:"Invoke Commands.vi"("Command Params"=w652, "Function Name"=w654) -> ("Params"=w651:u8, "Started"=w646:bool)  [unwired: 7 in, 1 out]
        n422 = Array Subset(array=w652, length (row)=w651) -> (w650:string[][])  [unwired: 3 in]
        n423 = Select(t="Executing" ("Cmd Status"), s=w646, f="" ("Cmd Status")) -> (s? t:f=w647:string)
        n424 = local write "Cmd Status"(w647) -> ()
      }
      event "CheckList": Double Click {
        # "Shift clears all"
        # "Update symbols on the listbox"
        n425 = event-data() -> ("PlatMods.Shift"=w658:bool, "Row"=w660:i32)  [unwired: 1 in]
        n426 = case shown="True" w658 {
          tunnel: w660 -> [w664 _]
          tunnel: 1 -> [w663 _]
          frame False {
            n427 = property on="CheckList" class="LstBox (strict)"() -> ("Item Symbols"=w662:i32[])  [unwired: 2 in, 2 out]
            n428 = Replace Array Subset(array=w662, new element=w663, index=w664) -> (w661:i32[])
            n429 = property on="CheckList" class="LstBox (strict)"("Item Symbols"=w661) -> ()  [unwired: 2 in, 2 out]
          }
          frame True {
            w665 = 0 ("Top Row")
            n430 = property on="CheckList" class="LstBox (strict)"() -> ("Number of Rows"=w667:u32)  [unwired: 2 in, 2 out]
            n431 = Initialize Array(0, w667) -> (w666:i32[])
            n432 = property on="CheckList" class="LstBox (strict)"("Top Row"=w665, "Value"=w665, "Item Symbols"=w666) -> ()  [unwired: 2 in, 2 out]
          }
        }
      }
      event "CheckList": Key Down {
        # "Update symbols on the listbox\nLeft and right keys check and uncheck"
        n433 = event-data() -> ("VKey"=w671:T21)  [unwired: 1 in]
        n434 = case shown="\"Left\", \"Right\"" w671 {
          selector: w671 -> [w676 _]
          tunnel: eventvkey."Left" ("VKey") -> [w674 _]
          frame "Left", "Right" {
            n435 = Equal?(x=w674, y=w676) -> (x = y?=w675:bool)
            n436 = Select(t=0, s=w675, f=1) -> (s? t:f=w677:i32)
            n437 = property on="CheckList" class="LstBox (strict)"() -> ("Item Symbols"=w680:i32[])  [unwired: 2 in, 2 out]
            n438 = Replace Array Subset(array=w680, new element=w677, index="CheckList") -> (w679:i32[])
            n439 = property on="CheckList" class="LstBox (strict)"("Item Symbols"=w679) -> ()  [unwired: 2 in, 2 out]
          }
          frame Default {
          }
        }
      }
      event "Motor.Enable": Value Change {
        # "When the test mode otor enable helper is set, update that\ntree row item's value"
        n440 = event-data() -> ("NewVal"=w686:bool)  [unwired: 1 in]
        n441 = Unbundle("Motor") -> ("Value"=w685:dbl)  [unwired: 1 out]
        n442 = Select(t=w685, s=w686, f=0.0) -> (s? t:f=w683:dbl)
        n443 = call <vilib>:"NT Write Number.vi"("Numeric"=w683, "Name"=w682) -> ()  [unwired: 9 in, 1 out]
      }
      event "Test Slider": Value Change {
        # "When the test mode slider helper is set, update that\ntree row item's value"
        n444 = event-data() -> ("NewVal"=w689:dbl)  [unwired: 1 in]
        n445 = call <vilib>:"NT Write Number.vi"("Numeric"=w689, "Name"=w690) -> ()  [unwired: 9 in, 1 out]
      }
      event "On/Off": Value Change {
        # "When the test mode on/off helper value is set, update that\ntree row item's value"
        n446 = event-data() -> ("NewVal"=w694:bool)  [unwired: 1 in]
        n447 = Boolean To (0,1)(Boolean=w694) -> (0, 1=w693:i16)
        n448 = call <vilib>:"NT Write Number.vi"("Numeric"=w693, "Name"=w692) -> ()  [unwired: 9 in, 1 out]
      }
      event "Rev/Fwd": Value Change {
        # "When the test mode helper value for relays is set, update that\ntree row item's value"
        n449 = event-data() -> ("NewVal.Forward"=w702:bool, "NewVal.Reverse"=w701:bool)  [unwired: 1 in]
        n450 = Boolean To (0,1)(Boolean=w702) -> (0, 1=w698:i16)
        n451 = Boolean To (0,1)(Boolean=w701) -> (0, 1=w700:i16)
        n452 = Negate(x=w700) -> (-x=w699:i16)
        n453 = Add(x=w698, y=w699) -> (x+y=w697:i16)
        n454 = call <vilib>:"NT Write Number.vi"("Numeric"=w697, "Name"=w696) -> ()  [unwired: 9 in, 1 out]
      }
      event "Test Ring": Value Change {
        # "When a test mode helper value is selected from the ring,\nset the tree item's variable to the string value"
        n455 = event-data() -> ("NewVal"=w706:u16)  [unwired: 1 in]
        n456 = property on="Test Ring" class="Ring (strict)"() -> ("Strings []"=w707:string[])  [unwired: 2 in, 2 out]
        n457 = Index Array(array=w707, index=w706) -> (element=w705:string)
        n458 = call <vilib>:"NT Write String.vi"("String"=w705, "Name"=w704) -> ()  [unwired: 9 in, 1 out]
      }
      event "Rec Mode": Value Change {
        # "Update globals for recording mode and path to read log from.\nClear when logging and let NetworkTables set path for vision to\nuse."
        n459 = event-data() -> ("NewVal"=w718:enum32{"Stop", "Record", "Playback"})  [unwired: 1 in]
        n460 = global write "WPI_DashboardLogging Global.vi" "Logging Filename"(path "") -> ()
        n461 = global write "WPI_DashboardLogging Global.vi" "Recording"(w718) -> ()
        n462 = case shown="\"Playback\"" w718 {
          tunnel: w717 -> [_ w720 w729]
          tunnel: [_ _ w728] -> w715
          tunnel: [_ _ w727] -> _
          tunnel: w713 -> [_ _ w725]
          tunnel: cluster{i32, i32} {-250, 170} -> [_ _ w724]
          tunnel: [_ _ T22 {"Image Size"=TRUE, "Image Type"=TRUE, "Pixel Value"=TRUE, "ROI Information"=TRUE, "Zoom Factor"=FALSE} ("Image Information Shown:All Elements")] -> w708
          tunnel: [_ _ TRUE ("Zoom Factor")] -> w709
          tunnel: w711 -> [_ _ w721]
          frame Default {
          }
          frame "Stop", "Record" {
            # "Place Window too"
            n463 = invoke class="VI" method="FP.Close"(reference=w720) -> (reference out=w719:refnum<vi>)  [unwired: 2 in, 2 out]
            n464 = invoke class="VI" method="Abort VI"(reference=w719) -> ()  [unwired: 2 in, 3 out]
          }
          frame "Playback" {
            n465 = call "Open Playback Panel.vi"("Offset"=w724, "DB VI Ref"=w725, "Playback in"=w729) -> ("Playback out"=w726:refnum<vi>)  [unwired: 8 in]
            n466 = register-events(w726, w721) -> (reference out=w728:refnum<event-registration>, error out=w727:errorcluster)  [unwired: 2 in]
          }
        }
        n467 = property on="Camera Image Right" class="ImageControl"("Image Information Shown"=w708, "Image Information Visible"=w709) -> ()  [unwired: 2 in, 2 out]
        n468 = property on="Camera Image" class="ImageControl"("Image Information Shown"=w708, "Image Information Visible"=w709) -> ()  [unwired: 2 in, 2 out]
        n469 = call <vilib>:"WPI_DashboardNT Log FieldName Cache.vi"("Operation"=enum16{"Lookup/Add", "Index", "Clear"}."Clear") -> ()  [unwired: 8 in, 3 out]
      }
      event Panel Close {
        w731 = enum32{"Stop", "Record", "Playback"}."Stop" ("Rec Mode")
        # "Playback window has been closed, abort"
        n470 = event-data() -> ()  [unwired: 1 in, 4 out]
        n471 = local write "Rec Mode"(w731) -> ()
        n472 = global write "WPI_DashboardLogging Global.vi" "Recording"(w731) -> ()
      }
      event Panel Close {
        # "Abort playback window and ourself"
        n473 = event-data() -> ()  [unwired: 1 in, 4 out]
        n474 = invoke class="VI" method="FP.Close"(reference=w735) -> (reference out=w734:refnum<vi>)  [unwired: 2 in, 2 out]
        n475 = invoke class="VI" method="Abort VI"(reference=w734) -> (error out=w733:errorcluster)  [unwired: 2 in, 2 out]
        n476 = invoke class="VI" method="Abort VI"(error in=w733) -> ()  [unwired: 2 in, 3 out]
      }
      event User Event {
        n477 = event-data() -> ("IDs"=w742:cluster{"RPC field ID":u16, "Unique ID":u16}, "String"=w741:string)  [unwired: 1 in]
        n478 = Bundle("IDs"=w742, "String"=w741) -> (w740:T12)  [unwired: 1 in]
        n479 = call <vilib>:"Retrieve RPC Response.vi"("RPC Response"=w740) -> ("Output"=w738:string[][])  [unwired: 10 in]
        n480 = Build Array (concatenate)(w736, w738) -> (w737:string[][])
        n481 = local write "Command Params"(w737) -> ()
        n482 = local write "Cmd Status"("" ("Cmd Status")) -> ()
      }
      event "Tree": Double Click {
        n483 = event-data() -> ("PlatMods"=w748:T25, "Tag"=w745:string)  [unwired: 1 in]
        n484 = Unbundle(w748) -> ("Shift"=w747:bool)  [unwired: 4 out]
        n485 = String Subset(string=w745, length (rest)=1 ("length (rest)")) -> (substring=w744:string)  [unwired: 1 in]
        n486 = Not(x=w747) -> (.not. x?=w746:bool)
        n487 = case shown="\"/\"" w744 {
          tunnel: w745 -> [_ w751]
          tunnel: w746 -> [_ w750]
          frame Default {
          }
          frame "/" {
            n488 = call <vilib>:"NT Update Persistence.vi"("Persistence"=w750, "Name"=w751) -> ()  [unwired: 9 in, 1 out]
          }
        }
      }
    }
  }
  n489 = while {
    tunnel: w62 -> [w753]
    i -> [w756]
    stop <- FALSE stop-if-true
    n490 = Wait (ms)(milliseconds to wait=u32 100) -> ()  [unwired: 1 out]
    n491 = case shown="\"Playback\"" "Rec Mode" {
      tunnel: w756 -> [_ _ w771]
      tunnel: [u32 2829099 ("Base Color") u32 11141120 ("Target Color") w760] -> w752
      frame "Stop", Default {
        # "Reset the color, extra updates don't cost much"
      }
      frame "Record" {
      }
      frame "Playback" {
        # "Playback"
        n492 = Quotient & Remainder(x=w771, y=u32 50 ("milliseconds to wait")) -> (x-y*floor(x/y)=w767:u32)  [unwired: 1 out]
        n493 = Divide(x=w767, y=u32 50 ("milliseconds to wait")) -> (x/y=w764:dbl)
        n494 = Multiply(x=6.283185307179586, y=w764) -> (x*y=w769:dbl)
        n495 = Sine(x=w769) -> (sin(x)=w768:dbl)
        n496 = Absolute Value(x=w768) -> (abs(x)=w761:dbl)
        n497 = call "Interpolate RGB Color.vi"("Proportion"=w761, "Target Color"=u32 30976, "Base Color"=u32 2829099) -> ("Result Color"=w760:u32)  [unwired: 8 in]
      }
    }
    n498 = property class="Pane"(reference=w753, "PaneColor"=w752) -> ()  [unwired: 1 in, 2 out]
  }
  n499 = property on="On/Off" class="Bool (strict)"("Visible"=w33) -> ()  [unwired: 2 in, 2 out]
  n500 = property on="Motor" class="Clust (strict)"("Visible"=w33) -> ()  [unwired: 2 in, 2 out]
  n501 = property on="Progress" class="Clust (strict)"("Visible"=w33) -> ()  [unwired: 2 in, 2 out]
  n502 = property on="Test Ring" class="Ring (strict)"("Visible"=w33) -> ()  [unwired: 2 in, 2 out]
  n503 = property on="Rev/Fwd" class="Clust (strict)"("Visible"=w33) -> ()  [unwired: 2 in, 2 out]
  n504 = local write "Command Selection"(u16 0 ("milliseconds to wait")) -> ()
  n505 = while {
    tunnel: u16 1741 ("timeout ms (25000)") -> [w773]
    stop <- FALSE stop-if-true
    n506 = TCP Create Listener(10:w773) -> (0:w772:errorcluster, 3:w774:refnum<k5>)  [unwired: 4 in, 1 out]
    n507 = case shown="No Error" w772 {
      selector: w772 -> [w776 _]
      tunnel: w774 -> [w777 _]
      frame No Error {
        n508 = while {
          tunnel: w777 -> [w780]
          tunnel: w776 -> [w779]
          stop <- FALSE stop-if-true
          n509 = TCP Wait On Listener(8:w779, 11:w780) -> (0:w781:errorcluster, 4:w782:refnum<k5>)  [unwired: 2 in, 3 out]
          n510 = local write "TCP"(w782) -> ()
          n511 = case shown="No Error" w781 {
            frame No Error {
            }
            frame Error {
              n512 = Wait (ms)(milliseconds to wait=u32 1000) -> ()  [unwired: 1 out]
            }
          }
        }
      }
      frame Error {
        n513 = Wait (ms)(milliseconds to wait=u32 1000) -> ()  [unwired: 1 out]
      }
    }
  }
  n514 = local write "Command Params"(string[][] [] ("Command Params")) -> ()
  n515 = global write "WPI_DashboardLogging Global.vi" "Recording"(w56) -> ()
  n516 = local write "Rec Mode"(w56) -> ()
